vi "main_control_v1.vi"() -> ()   [LabVIEW 2021]
uses:
  Addons/DAQ_Pulse_Gen/DAQ_Control_2.ctl
  Addons/DAQ_Pulse_Gen/DAQ_Control_1.ctl
  Ver_2/Config_File_Paths_v2.ctl
  Ver_2/ZI_Data_v2.ctl
  Addons/DAQ_Pulse_Gen/DAQ_Control_3 .ctl
  <vilib>/Utility/file.llb/Write Delimited Spreadsheet (DBL).vi
  <vilib>/gmath/NumericalOptimization/Nonlinear Curve Fit LM formula string.vi
  <vilib>/Utility/Data Type/NI_Data Type.lvlib
  <vilib>/Analysis/NI_AALPro.lvlib
  <vilib>/gmath/NI_Gmath.lvlib
panel:
  out "tomography rotation memory (priv)":cluster{"Time":dbl[], dbl[]}[](array[cluster])
  in  "pulses type (priv)":string[](array[string])=["None", "Y pi/2", "X pi/2"]
  in  "stop":bool
  in  "Tab Control":T1(tab)=enum."Run single FID"
  out "Config folder":string
  out "Chennel names\nare correct (?)":bool
  out "Channel map":map{string, i32}(c390)
  out "Pulses map [us]":map{string, dbl}(c390)
  out "Sampling data":T2={"Sample Numbers"=20000000, "Sample  Frequency (Hz)"=20000000}
  out "Resource Address":T3={"ZI Address"="DEV714", "VISA Keithley"="KEITHLEY"}
  in  "Run tomography":bool
  in  "Run single FID":bool
  in  "Save for tomography":bool
  in  "Save single sequence":bool
  out "Pulses chart":cluster{dbl[], dbl[]}[](graph)
  in  "Reset sequence":bool
  in  "Channel":u16(ring) items=["LD pump", "LD repump", "LD probe", "pulse X", "pulse Y", "pulse Z", "Keithley ARM", "Keithley TRIG", "Accqusition TRIG", "Nonlinear coil", "None"]
  in  "Add pulse advanced":bool
  in  "Physical channels":string[](array[string])
  in  "Add pulse":bool
  in  "Time [us]":dbl
  in  "Z pi/2":bool
  in  "Z pi":bool
  in  "Y pi/2":bool
  in  "Y pi":bool
  in  "X pi/2":bool
  in  "X pi":bool
  in  "Add pumping":bool
  in  "Pumping":T4(ring)
  in  "save":bool
  out "Rotation signal 3":cluster{"Time":dbl[], "Array":dbl[]}[](graph)
  out "w":dbl format="%#_3f"
  out "q":dbl format="%#_3f"
  out "g2":dbl format="%#_3f"
  out "g1":dbl format="%#_3f"
  out "C":dbl format="%#_3f"
  out "B":dbl format="%#_3f"
  out "A":dbl format="%#_3f"
  in  "Enum":T5(ring)
  in  "Fit model":bool
  out "Rotation signal":cluster{"Time":dbl[], dbl[]}(graph)
  out "Rotation spectrum":waveform(dbl)[](graph)
  out "Differential signal":cluster{"Time":dbl[], "X":dbl[]}[](graph)
  out "Intensity signal":cluster{"Time":dbl[], dbl[]}(graph)
  out "Polarimeter":dbl(knob) scale=-10.0..10.0
  in  "Run single FID 2":bool
  out "Progress":dbl(slide) scale=0.0..100.0
  in  "Number of repetition":u32=1 min=1 step=1
  in  "Signal in X or Y (?)":bool
  in  "Plot type":u16(ring) items=["None + [ None ]", "None + [ Y pi ]", "None + [ Z(pi/2)+Y(pi) ]", "Y pi/2 + [ None ]", "Y pi/2 + [ Y pi ]", "Y pi/2 + [ Z(pi/2)+Y(pi) ]", "X pi/2 + [ None ]", "X pi/2 + [ Y pi ]", "X pi/2 + [ Z(pi/2)+Y(pi) ]"]
  in  "Save raw data (?)":bool
  in  "Save CYCLOPS data (?)":bool
  out "Rotation signal":cluster{"Time":dbl[], dbl[]}(graph)
  in  "Run tomography 2":bool
  in  "Averaging":u8=1 min=1 step=1
  out "Differential signal":cluster{"Time":dbl[], "X":dbl[]}[](graph)
  out "Intensity signal":cluster{"Time":dbl[], dbl[]}(graph)
  out "Progress":dbl(slide) scale=0.0..100.0
  out "Rotation spectrum":waveform(dbl)[](graph)
  out "Rotation":cluster{"Time":dbl[], dbl[]}(graph)
  # "To change that tab you need to go to block diagram"
  # "Probing will be added during saving"
  # "X"
  # "Y"
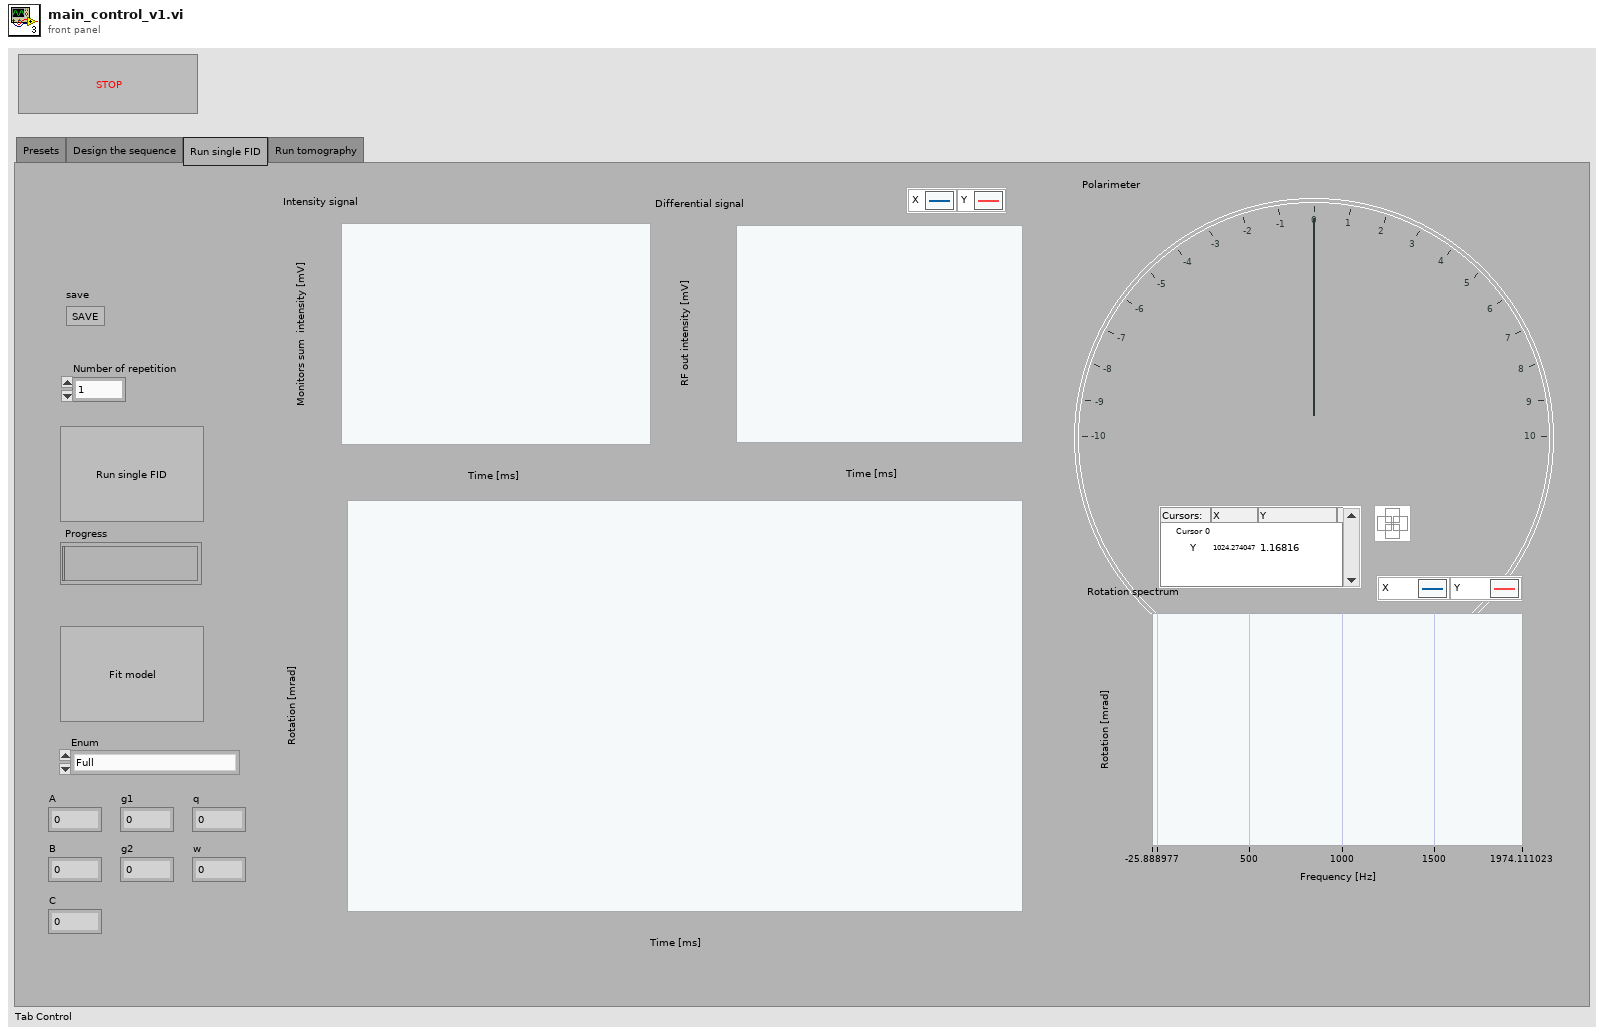
[diagram p1: front panel]
types:
  T1 = enum32{"Presets", "Design the sequence", "Run single FID", "Run tomography"}
  T2 = typedef "DAQ_Control_2.ctl" = cluster{"Sample Numbers":u32, "Sample  Frequency (Hz)":u32}
  T3 = cluster{"ZI Address":string, "VISA Keithley":refnum<visa-resource-name>}
  T4 = enum16{"Circular along X", "Linear in Y", "Linear in Z"}
  T5 = enum16{"Full", "A*Sin(w*t+q)*Exp(-g1*t)+C", "B*Exp(-q2*t)+C"}
  T6 = typedef "DAQ_Control_1.ctl" = cluster{"Port 2/line 6":cluster{"Timing 22":dbl[]}, "Port 2/line 5":cluster{"Timing 21":dbl[]}, "Port 2/line 4":cluster{"Timing 20":dbl[]}, "Port 2/line 3":cluster{"Timing 19":dbl[]}, "Port 2/line 2":cluster{"Timing 18":dbl[]}, "Port 2/line 1":cluster{"Timing 17":dbl[]}, "Port 2/line 0":cluster{"Timing 16":dbl[]}, "Port 1/line 7":cluster{"Timing 15":dbl[]}, "Port 1/line 6":cluster{"Timing 14":dbl[]}, "Port 1/line 5":cluster{"Timing 13":dbl[]}, "Port 1/line 4":cluster{"Timing 12":dbl[]}, "Port 1/line 3":cluster{"Timing 11":dbl[]}, "Port 1/line 2":cluster{"Timing 10":dbl[]}, "Port 1/line 1":cluster{"Timing 9":dbl[]}, "Port 1/line 0":cluster{"Timing 8":dbl[]}, "Port 0/line 7":cluster{"Timing 7\n":dbl[]}, "Port 0/line 6":cluster{"Timing 6\n":dbl[]}, "Port 0/line 5":cluster{"Timing 5\n":dbl[]}, "Port 0/line 4":cluster{"Timing 4\n":dbl[]}, "Port 0/line 3":cluster{"Timing 3\n":dbl[]}, "Port 0/line 2":cluster{"Timing 2":dbl[]}, "Port 0/line 1":cluster{"Timing 1\n":dbl[]}, "Port 0/line 0":cluster{"Timing 0":dbl[]}}
  T7 = typedef "Config_File_Paths_v2.ctl" = cluster{"ZI config file (.ini)":string, "Keithley config file (.ini)":string, "DAQ config file (.ini)":string}
  T8 = enum32{"Presets", "Design the sequence", "Run single FID"}
  T9 = enum8{"Enabled", "Disabled", "Disabled and Grayed Out"}
  T10 = cluster{"model":string, "Parameters":string[], "x":string}
  T11 = typedef "DAQ_Control_3 .ctl" = cluster{"Time Unit":enum16{"NanoSecond", "MicroSecond", "MilliSecond"}}
  T12 = typedef "ZI_Data_v2.ctl" = cluster{"R":dbl[], "Theta":dbl[], "X":dbl[], "Y":dbl[], "AuxIn0":dbl[], "AuxIn1":dbl[], "Frequency":dbl[], "DIO":dbl[], "Time":dbl[]}
  T13 = typedef "Resources_v2.ctl" = cluster{"ZI Handle":T14, "ZI ModHandle":T15, "VISA Keithley":refnum<visa-resource-name>}
  T14 = typedef "Zurich Instruments LabOne.lvlib/ziTypeHandle.ctl" = cluster{"handleValid":bool, "Conn":u64, "Path Prefix":string, "Handle":u64, "Connected":bool, "Clockbase(s)":dbl}
  T15 = typedef "Zurich Instruments LabOne.lvlib/ziTypeModHandle.ctl" = cluster{"handleValid":bool, "Conn":u64, "ModHandle":u64, "moduleID":string, "Path Prefix":string}
  T16 = typedef "Cutted_Data_v2.ctl" = cluster{"X":dbl[], "Y":dbl[], "Time":dbl[]}
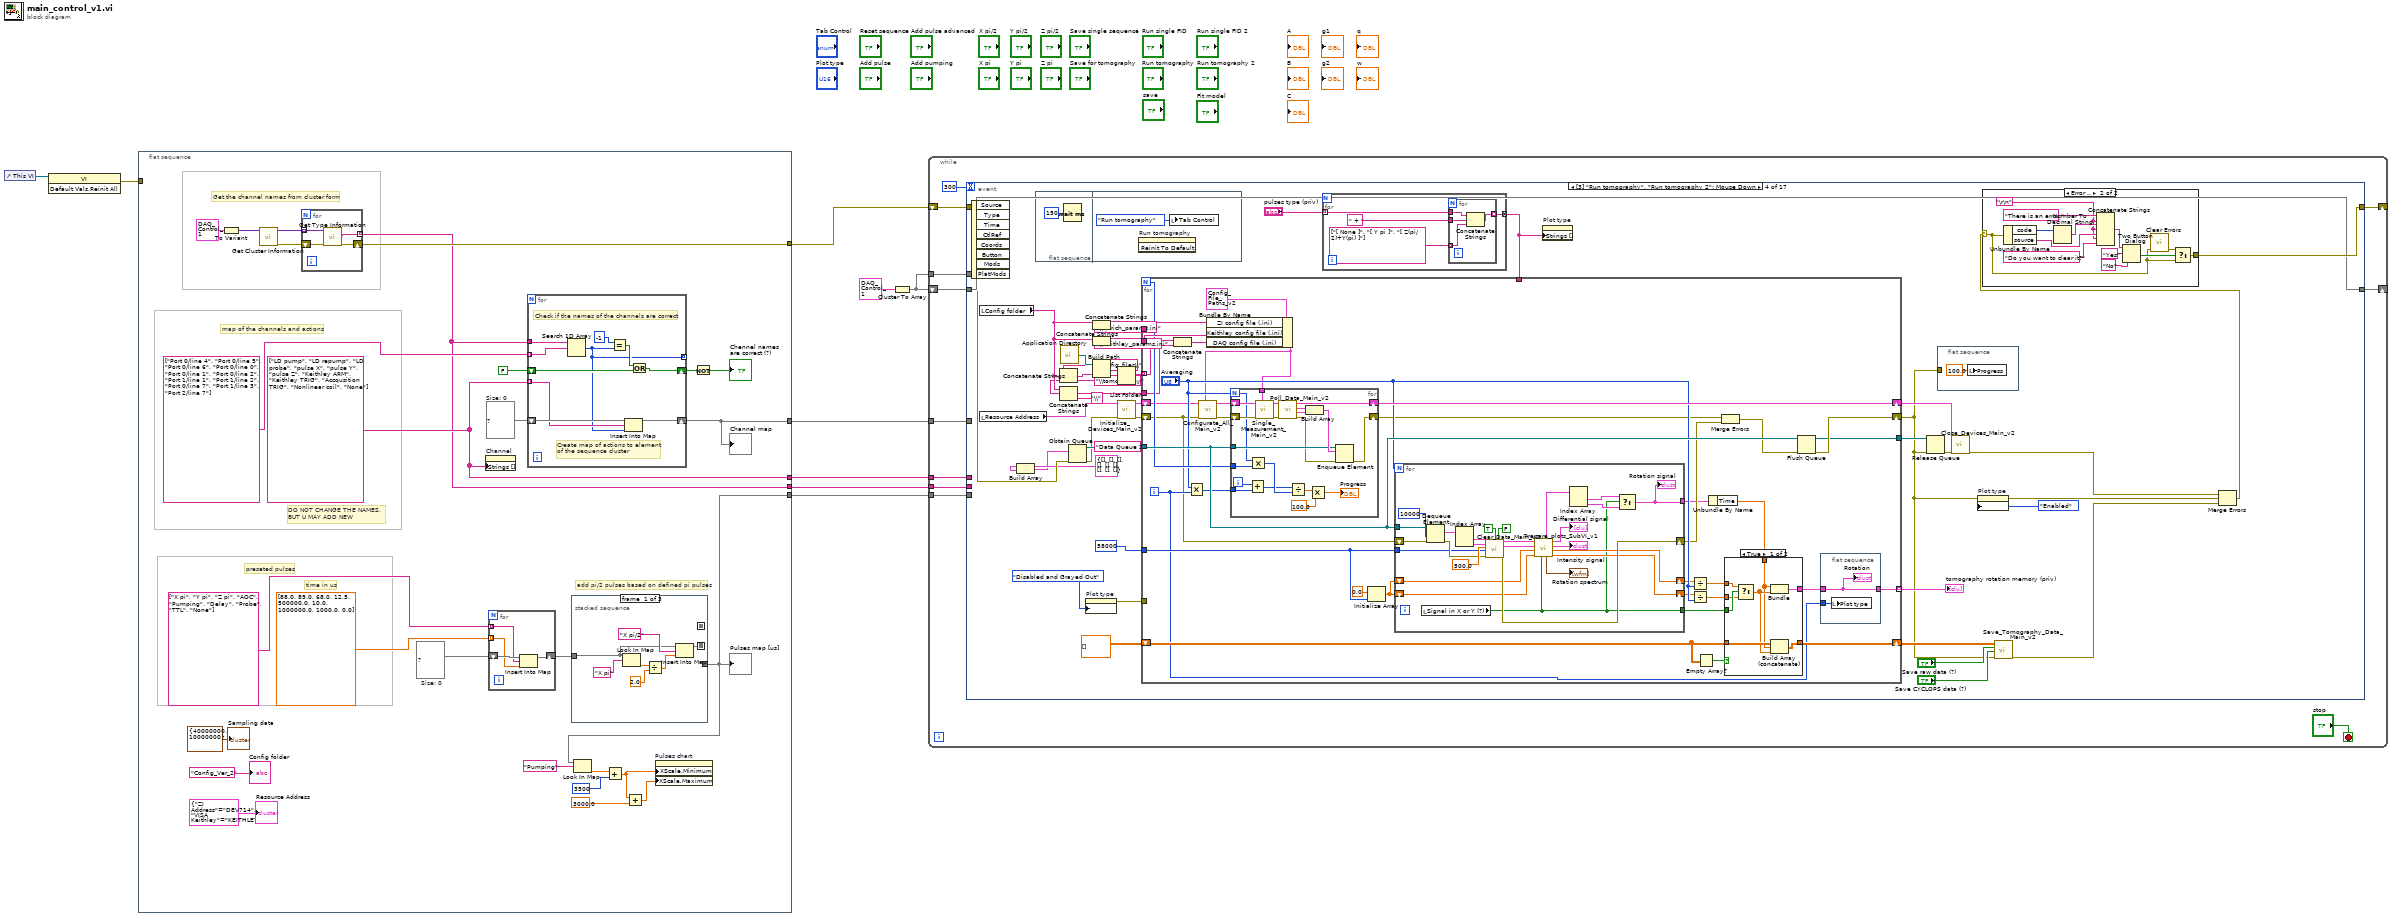
[diagram p0: block diagram]
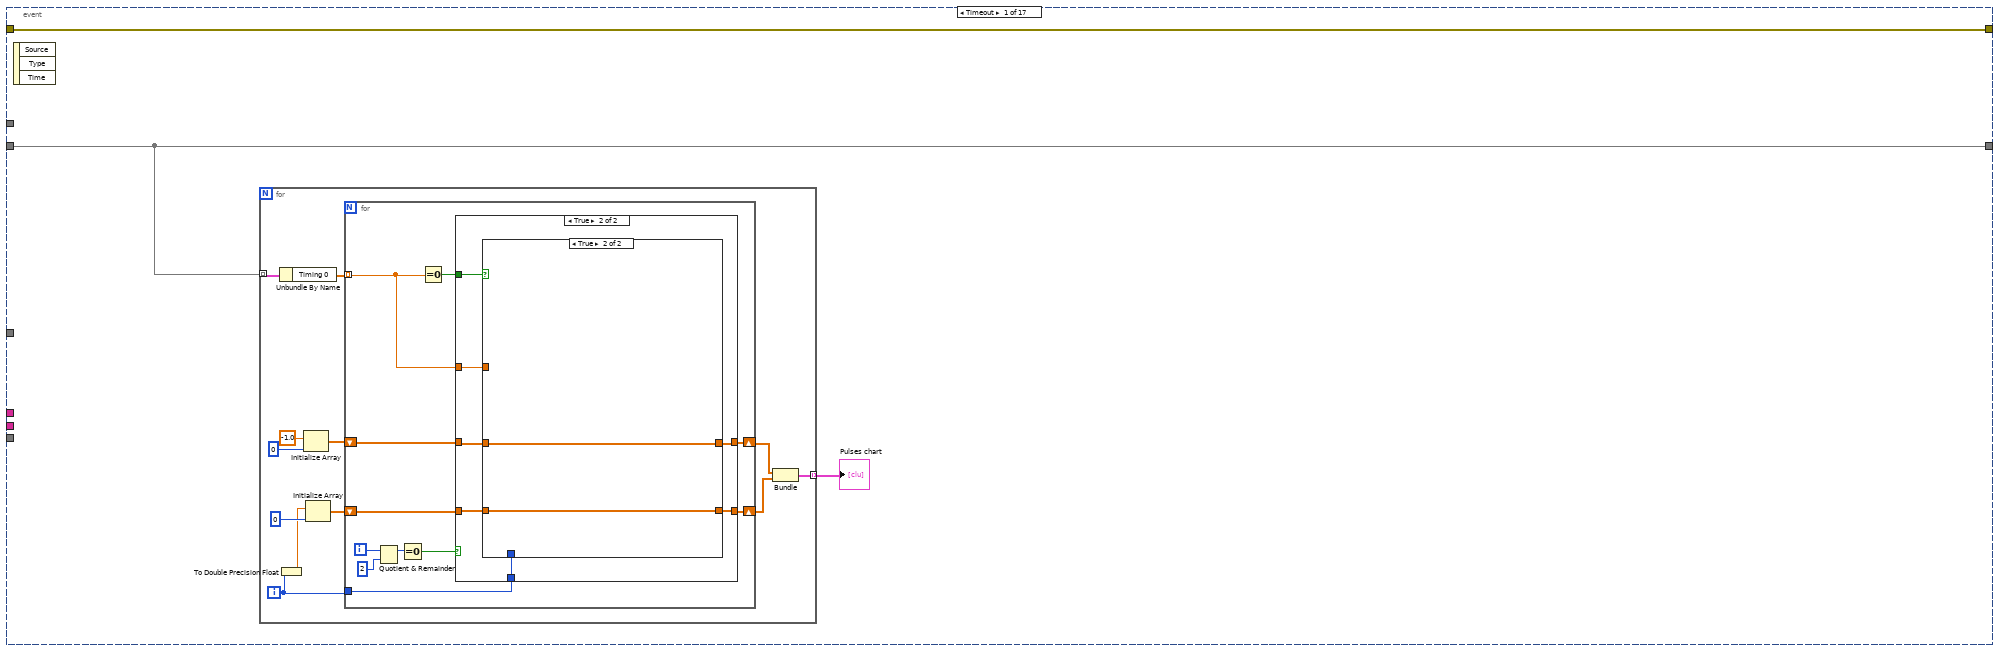
[diagram p2: hidden frame]
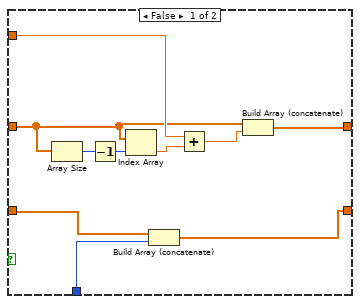
[diagram p3: hidden frame]
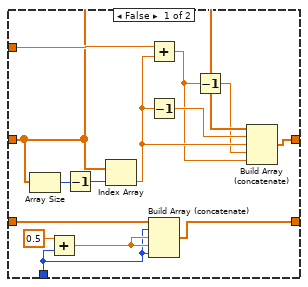
[diagram p4: hidden frame]
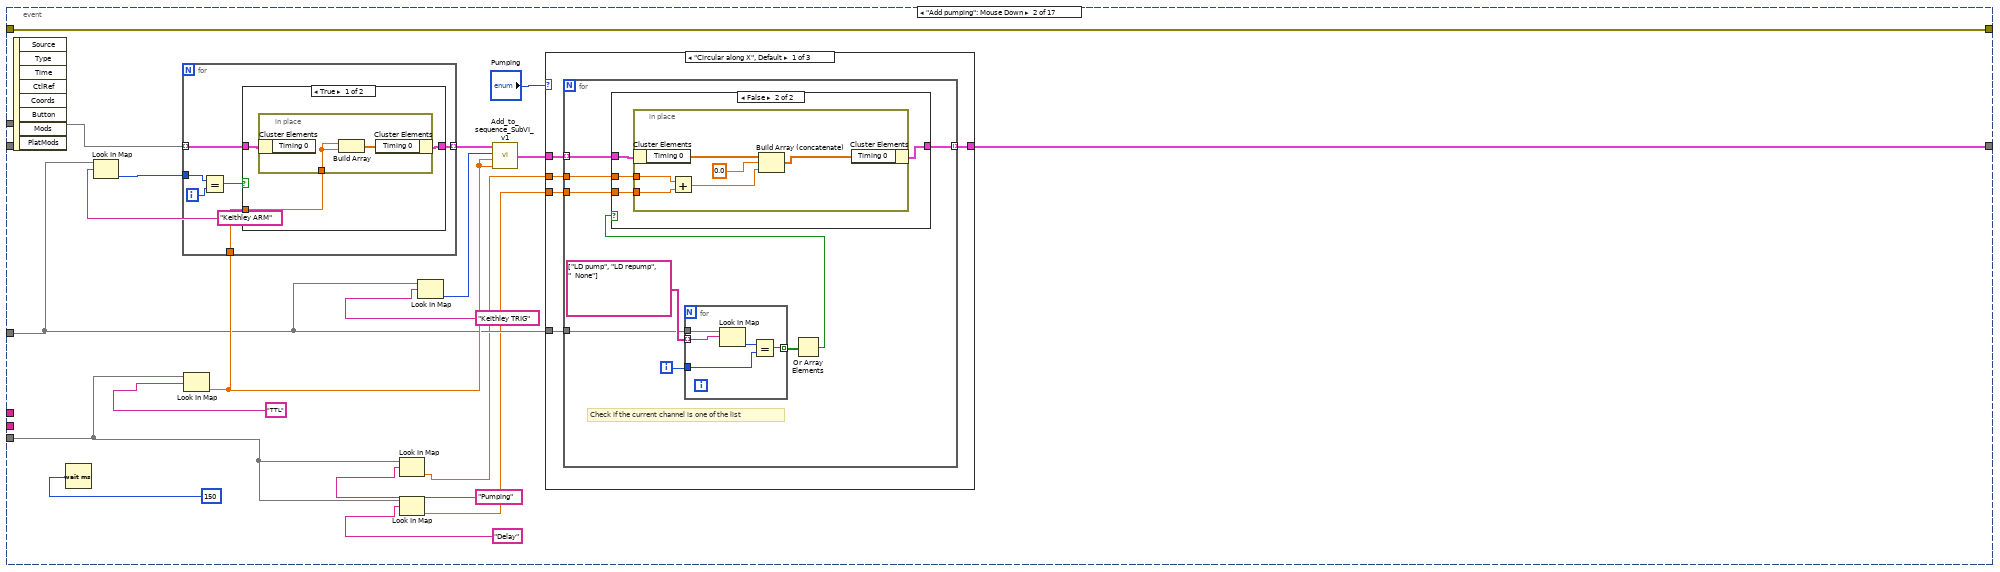
[diagram p5: hidden frame]
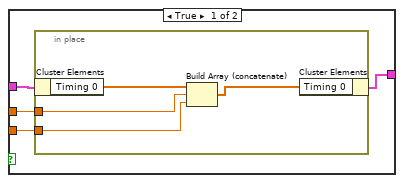
[diagram p6: hidden frame]
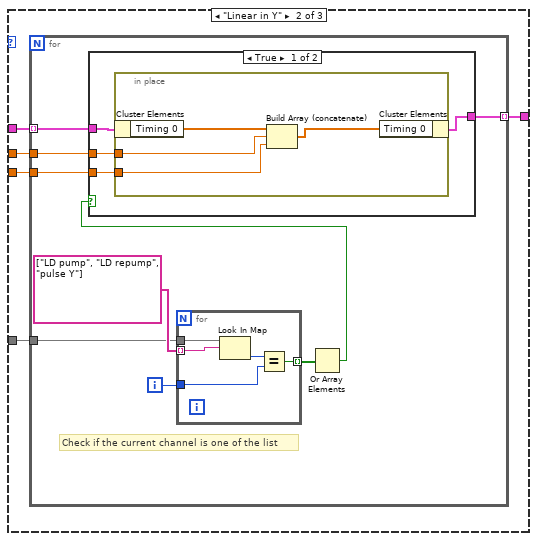
[diagram p7: hidden frame]
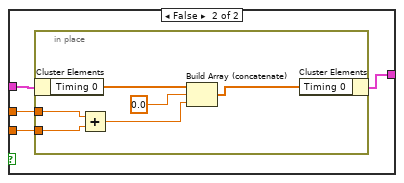
[diagram p8: hidden frame]
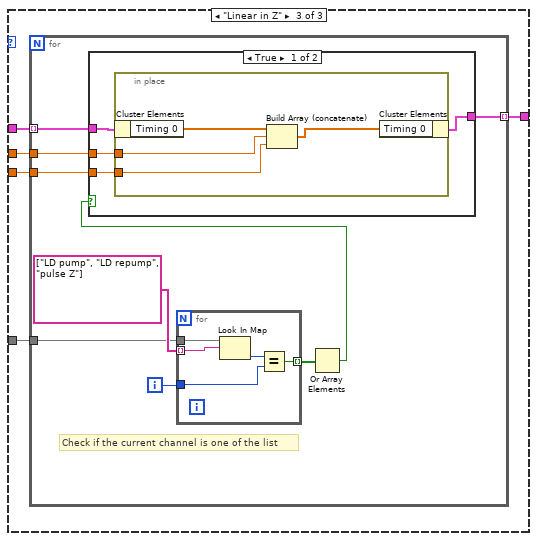
[diagram p9: hidden frame]
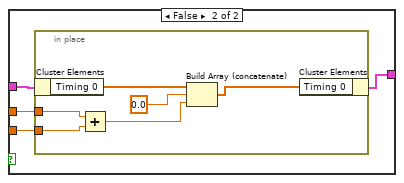
[diagram p10: hidden frame]
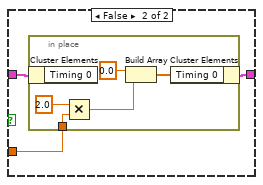
[diagram p11: hidden frame]
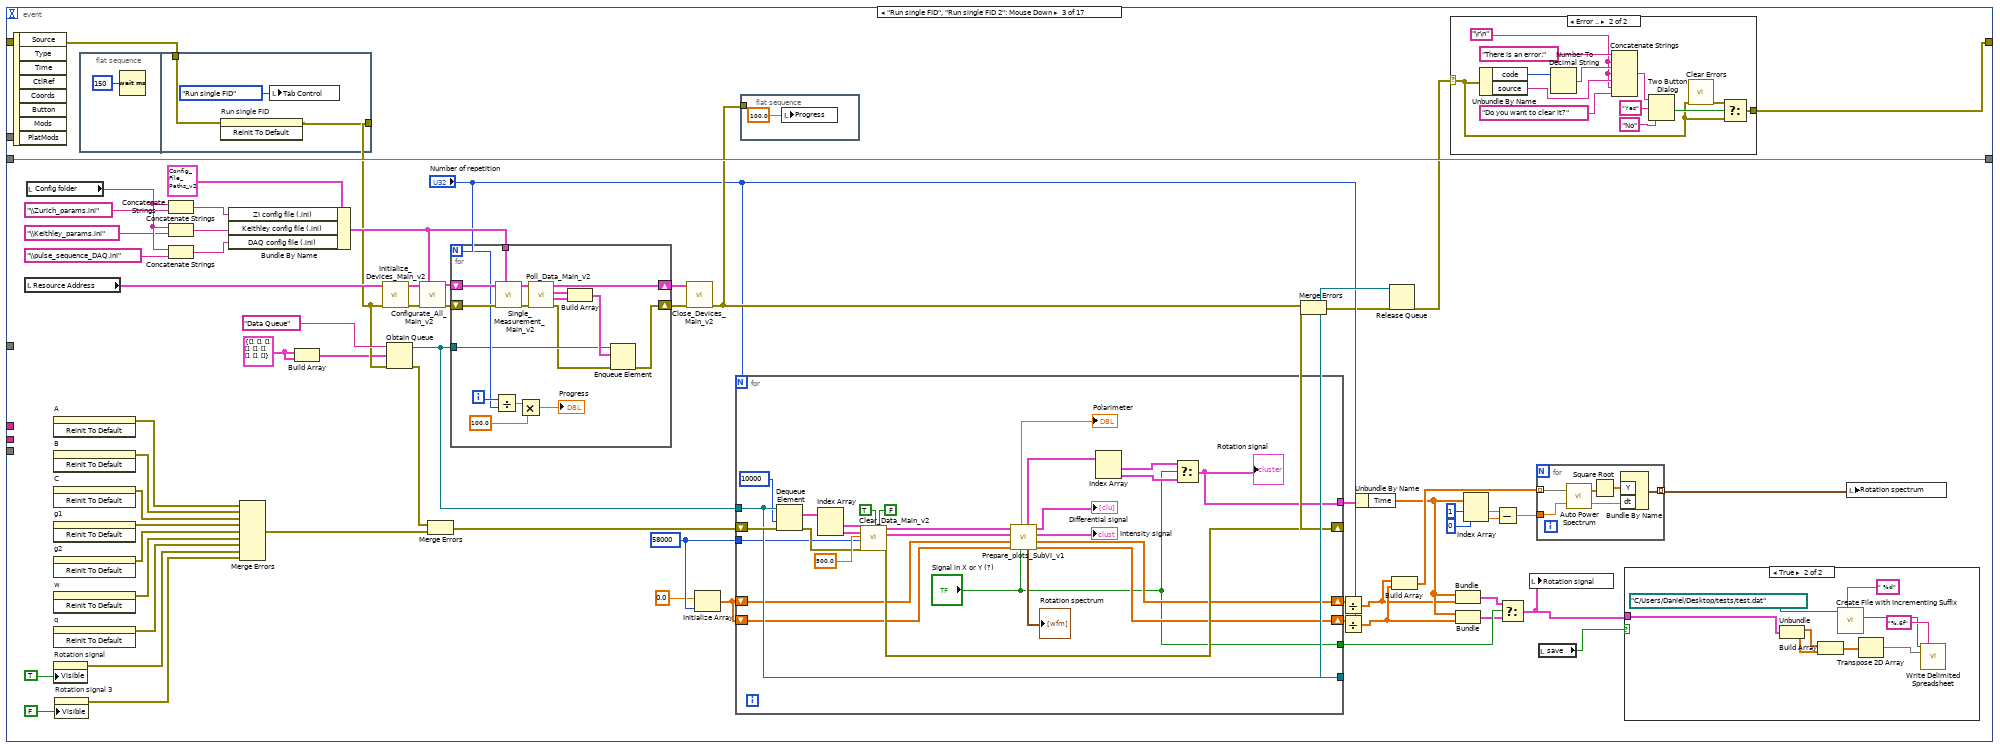
[diagram p12: hidden frame]
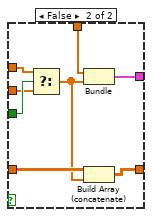
[diagram p15: hidden frame]
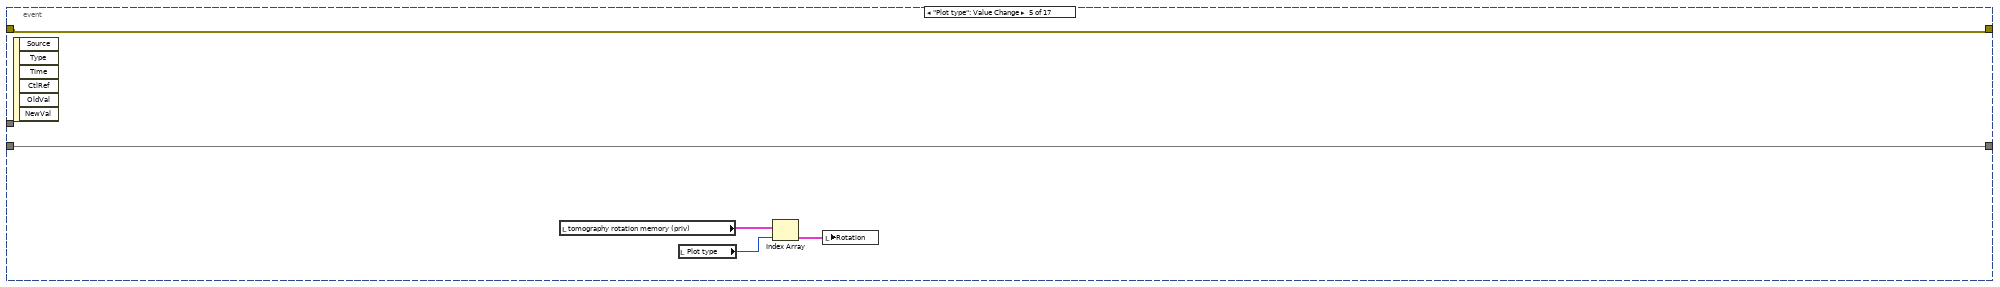
[diagram p17: hidden frame]
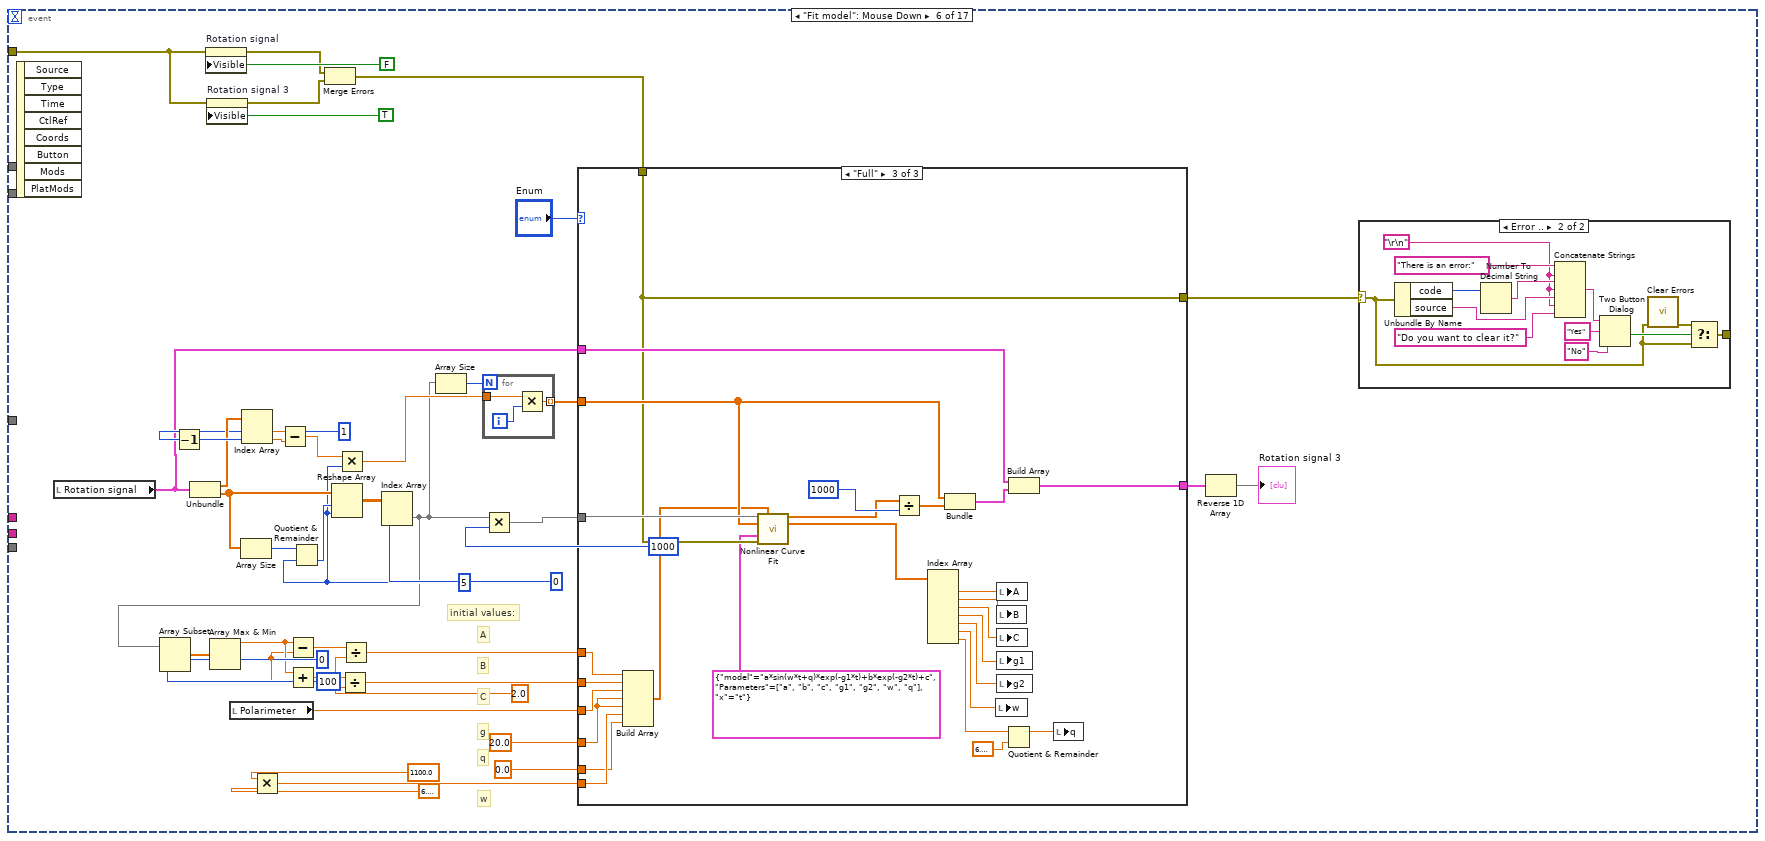
[diagram p18: hidden frame]
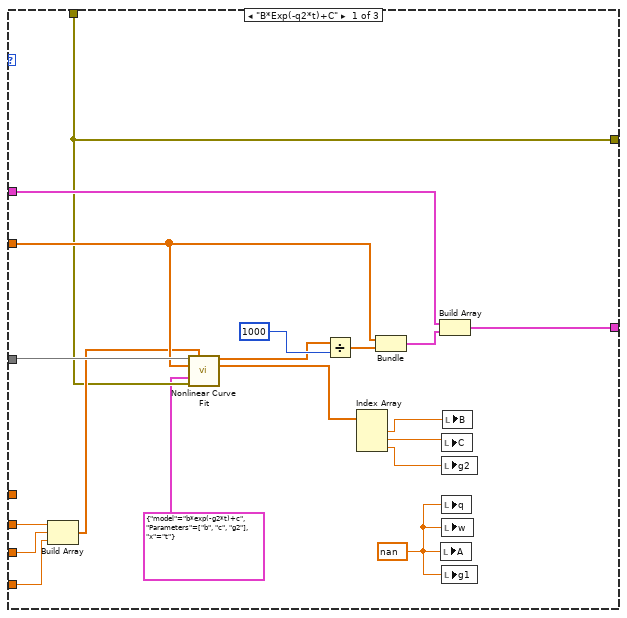
[diagram p20: hidden frame]
diagram:
  n1 = control-ref of="This VI"() -> (w2:refnum<vi>)
  n2 = invoke class="VI" method="Default Vals.Reinit All"(reference=w2) -> (error out=w1:errorcluster)  [unwired: 2 in, 2 out]
  n3 = flat-sequence {
    tunnel: [w23] -> w8
    tunnel: [w17] -> w7
    tunnel: [w22] -> w6
    tunnel: [w21] -> w5
    tunnel: [w20] -> w4
    tunnel: w1 -> [_]
    frame #0 {
      w27 = map{string, dbl} {}  # Size: 0
      w29 = map{string, i32} {}  # Size: 0
      w21 = string[] ["LD pump", "LD repump", "LD probe", "pulse X", "pulse Y", "pulse Z", "Keithley ARM", "Keithley TRIG", "Accqusition TRIG", "Nonlinear coil", "None"]
      # "DO NOT CHANGE THE NAMES,\nBUT U MAY ADD NEW"
      # "add pi/2 pulses based on defined pi pulses"
      # "preseted pulses"
      # "time in us"
      # "map of the channels and actions"
      # "Get the channel names from cluster form"
      n4 = To Variant(anything=T6 {"Port 2/line 6"={"Timing 22"=[]}, "Port 2/line 5"={"Timing 21"=[]}, "Port 2/line 4"={"Timing 20"=[]}, "Port 2/line 3"={"Timing 19"=[]}, "Port 2/line 2"={"Timing 18"=[]}, "Port 2/line 1"={"Timing 17"=[]}, "Port 2/line 0"={"Timing 16"=[]}, "Port 1/line 7"={"Timing 15"=[]}, "Port 1/line 6"={"Timing 14"=[]}, "Port 1/line 5"={"Timing 13"=[]}, "Port 1/line 4"={"Timing 12"=[]}, "Port 1/line 3"={"Timing 11"=[]}, "Port 1/line 2"={"Timing 10"=[]}, "Port 1/line 1"={"Timing 9"=[]}, "Port 1/line 0"={"Timing 8"=[]}, "Port 0/line 7"={"Timing 7\n"=[]}, "Port 0/line 6"={"Timing 6\n"=[]}, "Port 0/line 5"={"Timing 5\n"=[]}, "Port 0/line 4"={"Timing 4\n"=[]}, "Port 0/line 3"={"Timing 3\n"=[]}, "Port 0/line 2"={"Timing 2"=[]}, "Port 0/line 1"={"Timing 1\n"=[]}, "Port 0/line 0"={"Timing 0"=[]}} ("Sequence")) -> (Variant=w35:variant)
      n5 = call <vilib>:"Get Cluster Information.vi"("variant"=w35) -> ("error out"=w34:errorcluster, "cluster elements"=w33:variant[])  [unwired: 9 in]
      n6 = for {
        tunnel: w33 -> [w75] mode=indexing
        shift-right: [w73] -> w22
        shift-left: w34 -> [w74]
        tunnel: [w72] -> w20 mode=indexing
        n7 = call <vilib>:"Get Type Information.vi"("error in (no error)"=w74, "variant"=w75) -> ("error out"=w73:errorcluster, "name"=w72:string)  [unwired: 5 in, 3 out]
      }
      n8 = property on="Channel" class="Ring (strict)"("Strings []"=w21) -> ()  [unwired: 2 in, 2 out]
      n9 = for {
        shift-right: [w58] -> w24
        shift-left: w27 -> [w61]
        tunnel: string[] ["X pi", "Y pi", "Z pi", "AOC", "Pumping", "Delay", "Probe", "TTL", "None"] -> [w60] mode=indexing
        tunnel: dbl[] [88.0, 89.0, 68.0, 12.5, 500000.0, 10.0, 1000000.0, 1000.0, 0.0] -> [w59] mode=indexing
        n10 = Insert Into Map(map in=w61, key=w60, value=w59) -> (map out=w58:map{string, dbl})  [unwired: 2 out]
      }
      n11 = for {
        tunnel: w20 -> [w71]
        tunnel: string[] ["Port 0/line 4", "Port 0/line 5", "Port 0/line 6", "Port 0/line 0", "Port 0/line 1", "Port 0/line 2", "Port 1/line 1", "Port 1/line 2", "Port 0/line 7", "Port 1/line 3", "Port 2/line 7"] -> [w62] mode=indexing
        shift-right: [w67] -> w31
        shift-left: FALSE -> [w68]
        tunnel: [w64] -> _ mode=indexing
        shift-right: [w63] -> w23
        shift-left: w29 -> [w66]
        tunnel: w21 -> [w65] mode=indexing
        # "Create map of actions to element\nof the sequence cluster"
        # "Check if the names of the channels are correct"
        n12 = Search 1D Array(1D array=w71, element=w62) -> (index of element=w64:i32)  [unwired: 1 in]
        n13 = Equal?(x=-1, y=w64) -> (x = y?=w69:bool)
        n14 = Insert Into Map(map in=w66, key=w65, value=w64) -> (map out=w63:map{string, i32})  [unwired: 2 out]
        n15 = Or(x=w69, y=w68) -> (x .or. y?=w67:bool)
      }
      "Channel map" <- w23
      n16 = stacked-sequence {
        seq-local: [w37 _ _] -> [_ w44 _]
        seq-local: [_ w45 _] -> [_ _ w52]
        tunnel: w24 -> [w41 _ _]
        tunnel: [_ _ w51] -> w17
        frame #0 {
          n17 = Look In Map(map=w41, key="X pi") -> (value=w39:dbl)  [unwired: 1 in, 1 out]
          n18 = Divide(x=w39, y=2.0) -> (x/y=w40:dbl)
          n19 = Insert Into Map(map in=w41, key="X pi/2", value=w40) -> (map out=w37:map{string, dbl})  [unwired: 2 out]
        }
        frame #1 {
          n20 = Look In Map(map=w44, key="Y pi") -> (value=w50:dbl)  [unwired: 1 in, 1 out]
          n21 = Divide(x=w50, y=2.0) -> (x/y=w49:dbl)
          n22 = Insert Into Map(map in=w44, key="Y pi/2", value=w49) -> (map out=w45:map{string, dbl})  [unwired: 2 out]
        }
        frame #2 {
          n23 = Look In Map(map=w52, key="Z pi") -> (value=w54:dbl)  [unwired: 1 in, 1 out]
          n24 = Divide(x=w54, y=2.0) -> (x/y=w55:dbl)
          n25 = Insert Into Map(map in=w52, key="Z pi/2", value=w55) -> (map out=w51:map{string, dbl})  [unwired: 2 out]
        }
      }
      "Pulses map [us]" <- w17
      n26 = Look In Map(map=w17, key="Pumping") -> (value=w19:dbl)  [unwired: 1 in, 1 out]
      n27 = Add(x=w19, y=3500) -> (x+y=w16:dbl)
      n28 = Add(x=w16, y=3000.0) -> (x+y=w14:dbl)
      n29 = property on="Pulses chart" class="XYGraph (strict)"("XScale.Minimum"=w16, "XScale.Maximum"=w14) -> ()  [unwired: 2 in, 2 out]
      n30 = Not(x=w31) -> (.not. x?=→"Chennel names\nare correct (?)":bool)
      "Sampling data" <- T2 {"Sample Numbers"=40000000, "Sample  Frequency (Hz)"=10000000} ("Sampling data")
      "Config folder" <- "Config_Ver_2" ("Filename (ini)")
      "Resource Address" <- T3 {"ZI Address"="DEV714", "VISA Keithley"="KEITHLEY"} ("Resource Address")
    }
  }
  n31 = Cluster To Array(cluster=T6 {"Port 2/line 6"={"Timing 22"=[]}, "Port 2/line 5"={"Timing 21"=[]}, "Port 2/line 4"={"Timing 20"=[]}, "Port 2/line 3"={"Timing 19"=[]}, "Port 2/line 2"={"Timing 18"=[]}, "Port 2/line 1"={"Timing 17"=[]}, "Port 2/line 0"={"Timing 16"=[]}, "Port 1/line 7"={"Timing 15"=[]}, "Port 1/line 6"={"Timing 14"=[]}, "Port 1/line 5"={"Timing 13"=[]}, "Port 1/line 4"={"Timing 12"=[]}, "Port 1/line 3"={"Timing 11"=[]}, "Port 1/line 2"={"Timing 10"=[]}, "Port 1/line 1"={"Timing 9"=[]}, "Port 1/line 0"={"Timing 8"=[]}, "Port 0/line 7"={"Timing 7\n"=[]}, "Port 0/line 6"={"Timing 6\n"=[]}, "Port 0/line 5"={"Timing 5\n"=[]}, "Port 0/line 4"={"Timing 4\n"=[]}, "Port 0/line 3"={"Timing 3\n"=[]}, "Port 0/line 2"={"Timing 2"=[]}, "Port 0/line 1"={"Timing 1\n"=[]}, "Port 0/line 0"={"Timing 0"=[]}} ("Sequence")) -> (array=w3:cluster{"Timing 0":dbl[]}[])
  n32 = while {
    shift-right: [w77] -> _
    shift-left: w3 -> [w86]
    tunnel: w8 -> [w85]
    tunnel: w7 -> [w76]
    shift-right: [w81] -> _
    shift-left: w6 -> [w82]
    tunnel: w5 -> [w80]
    tunnel: w4 -> [w79]
    tunnel: w3 -> [w78]
    stop <- "stop" stop-if-true
    n33 = event shown="[3] \"Run tomography\", \"Run tomography 2\": Mouse Down" {
      selector: _ -> [_ _ _ _ _ _ _ _ _ _ _ _ _ _ _ _ _]
      dyn-events: _ -> [_ _ _ _ _ _ _ _ _ _ _ _ _ _ _ _ _]
      timeout: 300 -> [_ _ _ _ _ _ _ _ _ _ _ _ _ _ _ _ _]
      tunnel: w86 -> [w89 _ w343 w472 w608 _ w750 w762 w774 w786 w798 w810 w822 w845 w884 w955 _]
      tunnel: w85 -> [_ w151 _ _ _ _ w757 w769 w781 w793 w805 w817 w828 _ w897 w960 _]
      tunnel: w76 -> [_ w150 _ _ _ _ w751 w763 w775 w787 w799 w811 w823 w837 w894 w959 _]
      tunnel: [w89 w148 w343 w472 w608 _ w749 w761 w773 w785 w797 w809 w821 w834 w884 w955 w1097] -> w77
      tunnel: w82 -> [w88 w164 w342 w466 w609 w651 w753 w765 w777 w789 w801 w813 w826 w841 w879 w953 w1098]
      tunnel: [w88 w164 w321 w476 w609 _ w753 w765 w777 w789 w801 w813 w826 w841 w878 w952 w1098] -> w81
      tunnel: w80 -> [_ _ _ _ _ _ _ _ _ _ _ _ w829 _ _ _ _]
      tunnel: w79 -> [_ _ _ _ _ _ _ _ _ _ _ _ _ w843 _ _ _]
      tunnel: w78 -> [_ w147 _ _ _ _ _ _ _ _ _ _ _ _ _ _ w1097]
      event Timeout {
        n34 = event-data() -> ()  [unwired: 1 in, 3 out]
        n35 = for {
          tunnel: w89 -> [w101] mode=indexing
          tunnel: [w90] -> w87 mode=indexing
          i -> [w93]
          n36 = To Double Precision Float(number=w93) -> (double precision float=w97:dbl)
          n37 = Unbundle By Name(w101) -> ("Timing 0"=w100:dbl[])
          n38 = Initialize Array(-1.0 ("element"), 0 ("dimension size")) -> (w94:dbl[])
          n39 = Initialize Array(w97, 0 ("dimension size")) -> (w98:dbl[])
          n40 = for {
            tunnel: w100 -> [w103] mode=indexing
            shift-right: [w105] -> w91
            shift-left: w98 -> [w104]
            shift-right: [w107] -> w92
            shift-left: w94 -> [w106]
            tunnel: w93 -> [w102]
            i -> [w112]
            n41 = Quotient & Remainder(x=w112, y=2) -> (x-y*floor(x/y)=w110:i32)  [unwired: 1 out]
            n42 = Equal To 0?(x=w110) -> (x = 0?=w109:bool)
            n43 = Equal To 0?(x=w103) -> (x = 0?=w108:bool)
            n44 = case shown="True" w109 {
              tunnel: w108 -> [_ w129]
              tunnel: [w113 w128] -> w107
              tunnel: w106 -> [w115 w127]
              tunnel: [w120 w126] -> w105
              tunnel: w104 -> [w121 w125]
              tunnel: w103 -> [w116 w124]
              tunnel: w102 -> [w122 w123]
              frame False {
                n45 = Array Size(array=w115) -> (size(s)=w119:i32)
                n46 = Decrement(x=w119) -> (x-1=w118:i32)
                n47 = Index Array(array=w115, index=w118) -> (element=w117:dbl)
                n48 = Build Array (concatenate)(w121, w122) -> (w120:dbl[])
                n49 = Add(x=w116, y=w117) -> (x+y=w114:dbl)
                n50 = Build Array (concatenate)(w115, w114) -> (w113:dbl[])
              }
              frame True {
                n51 = case shown="True" w129 {
                  tunnel: [w140 w145] -> w128
                  tunnel: w127 -> [w134 w145]
                  tunnel: [w136 w144] -> w126
                  tunnel: w125 -> [w143 w144]
                  tunnel: w124 -> [w141 _]
                  tunnel: w123 -> [w137 _]
                  frame False {
                    n52 = Array Size(array=w134) -> (size(s)=w142:i32)
                    n53 = Add(x=0.5, y=w137) -> (x+y=w138:dbl)
                    n54 = Decrement(x=w142) -> (x-1=w135:i32)
                    n55 = Index Array(array=w134, index=w135) -> (element=w132:dbl)
                    n56 = Add(x=w141, y=w132) -> (x+y=w131:dbl)
                    n57 = Decrement(x=w132) -> (x-1=w133:dbl)
                    n58 = Build Array (concatenate)(w143, w137, w138, w138, w137) -> (w136:dbl[])
                    n59 = Decrement(x=w131) -> (x-1=w130:dbl)
                    n60 = Build Array (concatenate)(w134, w133, w132, w130, w131) -> (w140:dbl[])
                  }
                  frame True {
                  }
                }
              }
            }
          }
          n61 = Bundle(w92, w91) -> (w90:cluster{dbl[], dbl[]})  [unwired: 1 in]
        }
        "Pulses chart" <- w87
      }
      event "Add pumping": Mouse Down {
        n62 = event-data() -> ()  [unwired: 1 in, 8 out]
        n63 = Wait (ms)(milliseconds to wait=u32 150) -> ()  [unwired: 1 out]
        n64 = Look In Map(map=w151, key="Keithley ARM") -> (value=w161:i32)  [unwired: 1 in, 1 out]
        n65 = Look In Map(map=w150, key="TTL") -> (value=w156:dbl)  [unwired: 1 in, 1 out]
        n66 = for {
          tunnel: w147 -> [w278] mode=indexing
          tunnel: w161 -> [w280]
          tunnel: w156 -> [w277]
          tunnel: [w276] -> w159 mode=indexing
          i -> [w281]
          n67 = Equal?(x=w280, y=w281) -> (x = y?=w279:bool)
          n68 = case shown="True" w279 {
            tunnel: w278 -> [w284 w289]
            tunnel: w277 -> [w283 w288]
            tunnel: [w282 w287] -> w276
            frame True {
              n69 = in-place {
                in-place-border: w283 -> [w286]
                n70 = in-place-cluster #1(w284) -> ()  [unwired: 1 out]
                n71 = Build Array(w286, w286) -> (w285:dbl[])
                n72 = in-place-cluster #1("Timing 0"=w285) -> (w282:cluster{"Timing 0":dbl[]})
              }
            }
            frame False {
              n73 = in-place {
                in-place-border: w288 -> [w292]
                n74 = in-place-cluster #2(w289) -> ()  [unwired: 1 out]
                n75 = Multiply(x=2.0, y=w292) -> (x*y=w290:dbl)
                n76 = Build Array(0.0 ("element"), w290) -> (w294:dbl[])
                n77 = in-place-cluster #2("Timing 0"=w294) -> (w287:cluster{"Timing 0":dbl[]})
              }
            }
          }
        }
        n78 = Look In Map(map=w150, key="Pumping") -> (value=w146:dbl)  [unwired: 1 in, 1 out]
        n79 = Look In Map(map=w150, key="Delay") -> (value=w149:dbl)  [unwired: 1 in, 1 out]
        n80 = Look In Map(map=w151, key="Keithley TRIG") -> (value=w157:i32)  [unwired: 1 in, 1 out]
        n81 = call "Add_to_sequence_SubVI_v1.vi"("Delay [us]"=w156, "Pulse length [us]"=w156, "Channel number"=w157, "Array sequence in"=w159) -> ("Array sequence out"=w154:cluster{"Timing 0":dbl[]}[])
        n82 = case shown="\"Circular along X\", Default" "Pumping" {
          tunnel: w154 -> [w169 w206 w243]
          tunnel: w151 -> [w168 w205 w242]
          tunnel: w146 -> [w167 w204 w241]
          tunnel: w149 -> [w166 w203 w240]
          tunnel: [w165 w202 w239] -> w148
          frame "Circular along X", Default {
            n83 = for {
              tunnel: w169 -> [w173] mode=indexing
              tunnel: w168 -> [w175]
              tunnel: w167 -> [w172]
              tunnel: w166 -> [w171]
              tunnel: [w170] -> w165 mode=indexing
              i -> [w176]
              # "Check if the current channel is one of the list"
              n84 = for {
                tunnel: w175 -> [w200]
                tunnel: w176 -> [w199]
                tunnel: [w198] -> w178 mode=indexing
                tunnel: string[] ["LD pump", "LD repump", "  None"] -> [w197] mode=indexing
                n85 = Look In Map(map=w200, key=w197) -> (value=w201:i32)  [unwired: 1 in, 1 out]
                n86 = Equal?(x=w201, y=w199) -> (x = y?=w198:bool)
              }
              n87 = Or Array Elements(Boolean array=w178) -> (logical OR=w174:bool)
              n88 = case shown="False" w174 {
                tunnel: w173 -> [w182 w190]
                tunnel: w172 -> [w181 w189]
                tunnel: w171 -> [w180 w188]
                tunnel: [w179 w187] -> w170
                frame True {
                  n89 = in-place {
                    in-place-border: w181 -> [w185]
                    in-place-border: w180 -> [w184]
                    n90 = in-place-cluster #3(w182) -> ("Timing 0"=w186:dbl[])
                    n91 = Build Array (concatenate)(w186, w185, w184) -> (w183:dbl[])
                    n92 = in-place-cluster #3("Timing 0"=w183) -> (w179:cluster{"Timing 0":dbl[]})
                  }
                }
                frame False {
                  n93 = in-place {
                    in-place-border: w189 -> [w194]
                    in-place-border: w188 -> [w193]
                    n94 = in-place-cluster #4(w190) -> ("Timing 0"=w196:dbl[])
                    n95 = Add(x=w194, y=w193) -> (x+y=w192:dbl)
                    n96 = Build Array (concatenate)(w196, 0.0 ("element"), w192) -> (w195:dbl[])
                    n97 = in-place-cluster #4("Timing 0"=w195) -> (w187:cluster{"Timing 0":dbl[]})
                  }
                }
              }
            }
          }
          frame "Linear in Y" {
            n98 = for {
              tunnel: w206 -> [w210] mode=indexing
              tunnel: w205 -> [w212]
              tunnel: w204 -> [w209]
              tunnel: w203 -> [w208]
              tunnel: [w207] -> w202 mode=indexing
              i -> [w213]
              # "Check if the current channel is one of the list"
              n99 = for {
                tunnel: w212 -> [w237]
                tunnel: w213 -> [w236]
                tunnel: [w235] -> w215 mode=indexing
                tunnel: string[] ["LD pump", "LD repump", "pulse Y"] -> [w234] mode=indexing
                n100 = Look In Map(map=w237, key=w234) -> (value=w238:i32)  [unwired: 1 in, 1 out]
                n101 = Equal?(x=w238, y=w236) -> (x = y?=w235:bool)
              }
              n102 = Or Array Elements(Boolean array=w215) -> (logical OR=w211:bool)
              n103 = case shown="True" w211 {
                tunnel: w210 -> [w219 w227]
                tunnel: w209 -> [w218 w226]
                tunnel: w208 -> [w217 w225]
                tunnel: [w216 w224] -> w207
                frame True {
                  n104 = in-place {
                    in-place-border: w218 -> [w222]
                    in-place-border: w217 -> [w221]
                    n105 = in-place-cluster #5(w219) -> ("Timing 0"=w223:dbl[])
                    n106 = Build Array (concatenate)(w223, w222, w221) -> (w220:dbl[])
                    n107 = in-place-cluster #5("Timing 0"=w220) -> (w216:cluster{"Timing 0":dbl[]})
                  }
                }
                frame False {
                  n108 = in-place {
                    in-place-border: w226 -> [w231]
                    in-place-border: w225 -> [w230]
                    n109 = in-place-cluster #6(w227) -> ("Timing 0"=w233:dbl[])
                    n110 = Add(x=w231, y=w230) -> (x+y=w229:dbl)
                    n111 = Build Array (concatenate)(w233, 0.0 ("element"), w229) -> (w232:dbl[])
                    n112 = in-place-cluster #6("Timing 0"=w232) -> (w224:cluster{"Timing 0":dbl[]})
                  }
                }
              }
            }
          }
          frame "Linear in Z" {
            n113 = for {
              tunnel: w243 -> [w247] mode=indexing
              tunnel: w242 -> [w249]
              tunnel: w241 -> [w246]
              tunnel: w240 -> [w245]
              tunnel: [w244] -> w239 mode=indexing
              i -> [w250]
              # "Check if the current channel is one of the list"
              n114 = for {
                tunnel: w249 -> [w274]
                tunnel: w250 -> [w273]
                tunnel: [w272] -> w252 mode=indexing
                tunnel: string[] ["LD pump", "LD repump", "pulse Z"] -> [w271] mode=indexing
                n115 = Look In Map(map=w274, key=w271) -> (value=w275:i32)  [unwired: 1 in, 1 out]
                n116 = Equal?(x=w275, y=w273) -> (x = y?=w272:bool)
              }
              n117 = Or Array Elements(Boolean array=w252) -> (logical OR=w248:bool)
              n118 = case shown="True" w248 {
                tunnel: w247 -> [w256 w264]
                tunnel: w246 -> [w255 w263]
                tunnel: w245 -> [w254 w262]
                tunnel: [w253 w261] -> w244
                frame True {
                  n119 = in-place {
                    in-place-border: w255 -> [w259]
                    in-place-border: w254 -> [w258]
                    n120 = in-place-cluster #7(w256) -> ("Timing 0"=w260:dbl[])
                    n121 = Build Array (concatenate)(w260, w259, w258) -> (w257:dbl[])
                    n122 = in-place-cluster #7("Timing 0"=w257) -> (w253:cluster{"Timing 0":dbl[]})
                  }
                }
                frame False {
                  n123 = in-place {
                    in-place-border: w263 -> [w268]
                    in-place-border: w262 -> [w267]
                    n124 = in-place-cluster #8(w264) -> ("Timing 0"=w270:dbl[])
                    n125 = Add(x=w268, y=w267) -> (x+y=w266:dbl)
                    n126 = Build Array (concatenate)(w270, 0.0 ("element"), w266) -> (w269:dbl[])
                    n127 = in-place-cluster #8("Timing 0"=w269) -> (w261:cluster{"Timing 0":dbl[]})
                  }
                }
              }
            }
          }
        }
      }
      event "Run single FID", "Run single FID 2": Mouse Down {
        w303 = T12 {"R"=[], "Theta"=[], "X"=[], "Y"=[], "AuxIn0"=[], "AuxIn1"=[], "Frequency"=[], "DIO"=[], "Time"=[]} ("ZI Data")
        w337 = u16 58000 ("Fixed Number Of Points")
        n128 = event-data() -> ()  [unwired: 1 in, 8 out]
        n129 = local read "Resource Address"() -> (w359:T3)
        n130 = local read "Config folder"() -> (w356:string)
        n131 = invoke on="A" class="DigNum (strict)" method="Reinit To Default"() -> (error out=w311:errorcluster)  [unwired: 3 in, 2 out]
        n132 = invoke on="B" class="DigNum (strict)" method="Reinit To Default"() -> (error out=w312:errorcluster)  [unwired: 3 in, 2 out]
        n133 = invoke on="C" class="DigNum (strict)" method="Reinit To Default"() -> (error out=w313:errorcluster)  [unwired: 3 in, 2 out]
        n134 = invoke on="g1" class="DigNum (strict)" method="Reinit To Default"() -> (error out=w314:errorcluster)  [unwired: 3 in, 2 out]
        n135 = invoke on="g2" class="DigNum (strict)" method="Reinit To Default"() -> (error out=w310:errorcluster)  [unwired: 3 in, 2 out]
        n136 = invoke on="w" class="DigNum (strict)" method="Reinit To Default"() -> (error out=w309:errorcluster)  [unwired: 3 in, 2 out]
        n137 = invoke on="q" class="DigNum (strict)" method="Reinit To Default"() -> (error out=w308:errorcluster)  [unwired: 3 in, 2 out]
        n138 = property on="Rotation signal" class="XYGraph (strict)"("Visible"=TRUE) -> (error out=w304:errorcluster)  [unwired: 2 in, 1 out]
        n139 = property on="Rotation signal 3" class="XYGraph (strict)"("Visible"=FALSE) -> (error out=w297:errorcluster)  [unwired: 2 in, 1 out]
        n140 = flat-sequence {
          tunnel: w342 -> [w436]
          tunnel: [w435] -> w340
          frame #0 {
            n141 = Wait (ms)(milliseconds to wait=u32 150) -> ()  [unwired: 1 out]
          }
          frame #1 {
            n142 = invoke on="Run single FID" class="Bool (strict)" method="Reinit To Default"(error in=w436) -> (error out=w435:errorcluster)  [unwired: 2 in, 2 out]
            n143 = local write "Tab Control"(T8."Run single FID" ("Tab Control")) -> ()
          }
        }
        n144 = Concatenate Strings(w356, "\\Zurich_params.ini" ("string")) -> (w349:string)
        n145 = Concatenate Strings(w356, "\\Keithley_params.ini" ("string")) -> (w351:string)
        n146 = Concatenate Strings(w356, "\\pulse_sequence_DAQ.ini" ("string")) -> (w350:string)
        n147 = Bundle By Name(cluster=T7 {"ZI config file (.ini)"="Config_Ver_2\\Zurich_params.ini", "Keithley config file (.ini)"="Config_Ver_2\\Keithley_params.ini", "DAQ config file (.ini)"="Config_Ver_2\\pulse_sequence_DAQ.ini"} ("Config files paths"), "ZI config file (.ini)"=w349, "Keithley config file (.ini)"=w351, "DAQ config file (.ini)"=w350) -> (w346:T7)
        n148 = Merge Errors(w311, w312, w313, w314, w310, w309, w308, w304, w297) -> (w307:errorcluster)
        n149 = Build Array(w303, w303) -> (w302:T12[])
        n150 = call "Initialize_Devices_Main_v2.vi"("error in"=w340, "Resource Address"=w359) -> ("error out"=w357:errorcluster, "Resources"=w358:T13)  [unwired: 8 in]
        n151 = Obtain Queue(name (unnamed)="Data Queue", element data type=w302, error in (no error)=w340) -> (queue out=w339:refnum<queue>, error out=w306:errorcluster)  [unwired: 2 in, 1 out]
        n152 = call "Configurate_All_Main_v2.vi"("Resources in"=w358, "Config files paths"=w346, "error in"=w357) -> ("Resources out"=w348:T13, "error out"=w347:errorcluster)  [unwired: 6 in, 5 out]
        n153 = Merge Errors(w306, w307) -> (w305:errorcluster)
        n154 = for {
          N: "Number of repetition" -> [w426]
          tunnel: w346 -> [w431]
          shift-right: [w430] -> w345
          shift-left: w348 -> [w433]
          shift-right: [w418] -> w344
          shift-left: w347 -> [w432]
          tunnel: w339 -> [w421]
          i -> [w427]
          n155 = Divide(x=w427, y=w426) -> (x/y=w424:dbl)
          n156 = call "Single_Measurement_Main_v2.vi"("Config files paths"=w431, "error in"=w432, "Resources in"=w433) -> ("error out"=w428:errorcluster, "Resources out"=w429:T13)  [unwired: 6 in, 1 out]
          n157 = Multiply(x=w424, y=100.0) -> (x*y=→"Progress":dbl)
          n158 = call "Poll_Data_Main_v2.vi"("error in"=w428, "Resources in"=w429) -> ("error out"=w419:errorcluster, "ZI Data 3"=w420:T12, "ZI Data 0"=w417:T12, "Resources out"=w430:T13)  [unwired: 6 in]
          n159 = Build Array(w417, w420) -> (w422:T12[])
          n160 = Enqueue Element(queue=w421, element=w422, error in (no error)=w419) -> (error out=w418:errorcluster)  [unwired: 1 in, 2 out]
        }
        n161 = call "Close_Devices_Main_v2.vi"("error in"=w344, "Resources"=w345) -> ("error out"=w322:errorcluster)  [unwired: 9 in]
        n162 = Initialize Array(0.0 ("element"), w337) -> (w335:dbl[])
        n163 = for {
          N: "Number of repetition" -> [_]
          tunnel: w339 -> [w410]
          shift-right: [w407] -> w301
          shift-left: w305 -> [w412]
          tunnel: [w410] -> w338
          shift-right: [w400] -> w318
          shift-left: w335 -> [w403]
          tunnel: w337 -> [w406]
          shift-right: [w401] -> w319
          shift-left: w335 -> [w402]
          tunnel: [w389] -> w334
          tunnel: ["Signal in X or Y (?)"] -> w333
          n164 = Dequeue Element(queue=w410, timeout in ms (-1)=10000, error in (no error)=w412) -> (element=w411:T12[], error out=w408:errorcluster)  [unwired: 2 out]
          n165 = Index Array(array=w411) -> (element #1=w391:T12, element #2=w409:T12)  [unwired: 2 in]
          n166 = call "Clear_Data_Main_v2.vi"("ZI Data 0"=w391, "ZI Data 3"=w409, "Time Of Collected Data (ms)"=500.0, 3:"Fixed Number Of Points"=w406, "error in"=w408, 10:"Fixed Number Of Points"=TRUE ("Fixed Number Of Points"), "Check Phase Mismatch"=FALSE) -> ("Cutted Data 0"=w405:T16, "Cutted Data 3"=w404:T16, "error out"=w407:errorcluster)  [unwired: 7 in, 3 out]
          n167 = call "Prepare_plots_SubVI_v1.vi"("Signal in X or Y (?)"="Signal in X or Y (?)", "Y rot avg in"=w402, "X rot avg in"=w403, "Cutted Data 3"=w404, "Cutted Data 0"=w405) -> ("Y rot avg out"=w401:dbl[], "X rot avg out"=w400:dbl[], "Monitor"=→"Intensity signal":cluster{"Time":dbl[], dbl[]}, "RF out"=→"Differential signal":cluster{"Time":dbl[], "Y":dbl[]}[], "Rotation spectrum"=→"Rotation spectrum":waveform(dbl)[], "Rotation"=w396:cluster{"Time":dbl[], dbl[]}[], "Polarimeter"=→"Polarimeter":dbl)
          n168 = Index Array(array=w396) -> (element #1=w395:cluster{"Time":dbl[], dbl[]}, element #2=w394:cluster{"Time":dbl[], dbl[]})  [unwired: 2 in]
          n169 = Select(t=w395, s="Signal in X or Y (?)", f=w394) -> (s? t:f=w389:cluster{"Time":dbl[], dbl[]})
          "Rotation signal" <- w389
        }
        n170 = flat-sequence {
          tunnel: w322 -> [_]
          frame #0 {
            n171 = local write "Progress"(100.0 ("Progress")) -> ()
          }
        }
        n172 = Merge Errors(w322, w301) -> (w300:errorcluster)
        n173 = Divide(x=w318, y="Number of repetition") -> (x/y=w316:dbl[])
        n174 = Divide(x=w319, y="Number of repetition") -> (x/y=w317:dbl[])
        n175 = Unbundle By Name(w334) -> ("Time"=w325:dbl[])
        n176 = Release Queue(queue=w338, error in (no error)=w300) -> (error out=w299:errorcluster)  [unwired: 1 in, 2 out]
        n177 = Build Array(w316, w317) -> (w326:dbl[][])
        n178 = case shown="Error .." w299 {
          selector: w299 -> [w369 w370]
          tunnel: [w369 w373] -> w321
          frame No Error {
          }
          frame Error {
            w378 = "\r\n"
            n179 = Unbundle By Name(w370) -> ("code"=w381:i32, "source"=w379:string)
            n180 = Number To Decimal String(number=w381) -> (decimal integer string=w380:string)  [unwired: 1 in]
            n181 = Concatenate Strings("There is an error:" ("string"), w378, w380, w378, w379, w378, "Do you want to clear it?" ("string")) -> (w374:string)
            n182 = Two Button Dialog(message=w374, 1:"No" ("F button name (\"Cancel\")"), 2:"Yes" ("T button name (\"OK\")")) -> (T button?=w372:bool)
            n183 = call <vilib>:"Clear Errors.vi"("error in (no error)"=w370) -> ("error out"=w371:errorcluster)  [unwired: 5 in, 1 out]
            n184 = Select(t=w371, s=w372, f=w370) -> (s? t:f=w373:errorcluster)
          }
        }
        n185 = Bundle("Time"=w325, w316) -> (w331:cluster{"Time":dbl[], dbl[]})  [unwired: 1 in]
        n186 = Bundle("Time"=w325, w317) -> (w332:cluster{"Time":dbl[], dbl[]})  [unwired: 1 in]
        n187 = Index Array(array=w325, index #1=1 ("index"), index #2=0 ("index")) -> (element #1=w329:dbl, element #2=w330:dbl)
        n188 = Subtract(x=w329, y=w330) -> (x-y=w324:dbl)
        n189 = Select(t=w331, s=w333, f=w332) -> (s? t:f=w295:cluster{"Time":dbl[], dbl[]})
        n190 = local write "Rotation signal"(w295) -> ()
        n191 = for {
          tunnel: w326 -> [w388] mode=indexing
          tunnel: [w386] -> w323 mode=indexing
          tunnel: w324 -> [w383]
          n192 = call <vilib>:"Auto Power Spectrum.vi"("dt"=w383, "Signal (V)"=w388) -> ("df"=w387:dbl, "Power Spectrum (V^2 rms)"=w385:dbl[])
          n193 = Square Root(x=w385) -> (sqrt(x)=w384:dbl[])
          n194 = Bundle By Name("Y"=w384, "dt"=w387) -> (w386:waveform(dbl))  [unwired: 1 in]
        }
        n195 = local read "save"() -> (w296:bool)
        n196 = case shown="True" w296 {
          tunnel: w295 -> [_ w368]
          frame False {
          }
          frame True {
            n197 = Unbundle(w368) -> ("Time"=w367:dbl[], w366:dbl[])
            n198 = Build Array(w367, w366) -> (w365:dbl[][])
            n199 = call <vilib>:"Create File with Incrementing Suffix.vi"("format string (\" (%d)\")"=" %d" ("format string (\" (%d)\")"), "file path"=path "C:/Users/Daniel/Desktop/tests/test.dat") -> ("actual path"=w362:path)  [unwired: 7 in, 2 out]
            n200 = Transpose 2D Array(2D array=w365) -> (transposed array=w364:dbl[][])
            n201 = call-poly <vilib>:"Write Delimited Spreadsheet.vi"("file path (dialog if empty)"=w362, "format (%.3f)"="%.6f", "2D data"=w364) -> ()  [unwired: 11 in, 2 out]
          }
        }
        n202 = local write "Rotation spectrum"(w323) -> ()
      }
      event "Run tomography", "Run tomography 2": Mouse Down {
        w446 = T12 {"R"=[], "Theta"=[], "X"=[], "Y"=[], "AuxIn0"=[], "AuxIn1"=[], "Frequency"=[], "DIO"=[], "Time"=[]} ("ZI Data")
        w441 = "\\tomography" ("string")
        n203 = event-data() -> ()  [unwired: 1 in, 8 out]
        n204 = local read "Config folder"() -> (w442:string)
        n205 = local read "Resource Address"() -> (w471:T3)
        n206 = Build Array(w446, w446) -> (w445:T12[])
        n207 = flat-sequence {
          frame #0 {
            n208 = Wait (ms)(milliseconds to wait=u32 150) -> ()  [unwired: 1 out]
          }
          frame #1 {
            n209 = invoke on="Run tomography" class="Bool (strict)" method="Reinit To Default"() -> ()  [unwired: 3 in, 3 out]
            n210 = local write "Tab Control"(T1."Run tomography" ("Tab Control")) -> ()
          }
        }
        n211 = Concatenate Strings("Config_files\\" ("string"), w442, w441) -> (w444:string)
        n212 = Concatenate Strings(w442, w441, "\\" ("string")) -> (w440:string)
        n213 = call <vilib>:"Application Directory.vi"() -> ("Application Directory"=w474:path)
        n214 = Obtain Queue(name (unnamed)="Data Queue 2", element data type=w445, error in (no error)=w466) -> (queue out=w468:refnum<queue>, error out=w465:errorcluster)  [unwired: 2 in, 1 out]
        n215 = property on="Plot type" class="Ring (strict)"("DisabledEnum"=T9."Disabled and Grayed Out" ("Disabled")) -> (error out=w452:errorcluster)  [unwired: 2 in, 1 out]
        n216 = Concatenate Strings(w442, "\\Zurich_params.ini" ("string")) -> (w477:string)
        n217 = Concatenate Strings(w442, "\\Keithley_params.ini" ("string")) -> (w478:string)
        n218 = Build Path(base path=w474, name or relative path=w444) -> (appended path=w475:path)
        n219 = List Folder(path=w475) -> (filenames=w473:string[])  [unwired: 3 in, 3 out]
        n220 = call "Initialize_Devices_Main_v2.vi"("error in"=w465, "Resource Address"=w471) -> ("error out"=w469:errorcluster, "Resources"=w470:T13)  [unwired: 8 in]
        n221 = for {
          tunnel: "pulses type (priv)" -> [w484] mode=indexing
          tunnel: [w482] -> w455 mode=concatenating
          n222 = for {
            tunnel: " + " ("string") -> [w489]
            tunnel: w484 -> [w488]
            tunnel: string[] ["[ None ]", "[ Y pi ]", "[ Z(pi/2)+Y(pi) ]"] -> [w487] mode=indexing
            tunnel: [w486] -> w482 mode=indexing
            n223 = Concatenate Strings(w488, w489, w487) -> (w486:string)
          }
        }
        n224 = for {
          N -> [w518]
          tunnel: w478 -> [w526]
          tunnel: w477 -> [w525]
          tunnel: w473 -> [w490] mode=indexing
          shift-right: [w521] -> w438
          shift-left: w469 -> [w496]
          tunnel: w468 -> [w522]
          shift-right: [w523] -> w464
          shift-left: w470 -> [w495]
          tunnel: u16 58000 ("Fixed Number Of Points") -> [w519]
          tunnel: [w520] -> w462
          shift-right: [w514] -> w459
          shift-left: dbl[][] [] -> [w515]
          tunnel: w455 -> [_]
          tunnel: [w511] -> w454 mode=indexing
          tunnel: w452 -> [_]
          tunnel: w440 -> [w492]
          i -> [w512]
          n225 = Concatenate Strings(w492, w490) -> (w491:string)
          n226 = Multiply(x="Averaging", y=w512) -> (x*y=w517:i32)
          n227 = Bundle By Name(cluster=T7 {"ZI config file (.ini)"="Config_Ver_2\\Zurich_params.ini", "Keithley config file (.ini)"="Config_Ver_2\\Keithley_params.ini", "DAQ config file (.ini)"="Config_Ver_2\\pulse_sequence_DAQ.ini"} ("Config files paths"), "ZI config file (.ini)"=w525, "Keithley config file (.ini)"=w526, "DAQ config file (.ini)"=w491) -> (w493:T7)
          n228 = call "Configurate_All_Main_v2.vi"("Resources in"=w495, "Config files paths"=w493, "error in"=w496) -> ("Resources out"=w494:T13, "error out"=w497:errorcluster)  [unwired: 6 in, 5 out]
          n229 = for {
            N: "Averaging" -> [w575]
            shift-right: [w587] -> w523
            shift-left: w494 -> [w589]
            shift-right: [w578] -> w509
            shift-left: w497 -> [w588]
            tunnel: w522 -> [w580]
            tunnel: w493 -> [w577]
            tunnel: w518 -> [w576]
            tunnel: w517 -> [w572]
            i -> [w573]
            n230 = Add(x=w573, y=w572) -> (x+y=w571:i32)
            n231 = Multiply(x=w575, y=w576) -> (x*y=w574:i32)
            n232 = call "Single_Measurement_Main_v2.vi"("Config files paths"=w577, "error in"=w588, "Resources in"=w589) -> ("error out"=w585:errorcluster, "Resources out"=w586:T13)  [unwired: 6 in, 1 out]
            n233 = call "Poll_Data_Main_v2.vi"("error in"=w585, "Resources in"=w586) -> ("error out"=w579:errorcluster, "ZI Data 3"=w582:T12, "ZI Data 0"=w569:T12, "Resources out"=w587:T13)  [unwired: 6 in]
            n234 = Divide(x=w571, y=w574) -> (x/y=w583:dbl)
            n235 = Build Array(w569, w582) -> (w581:T12[])
            n236 = Multiply(x=w583, y=100.0) -> (x*y=→"Progress":dbl)
            n237 = Enqueue Element(queue=w580, element=w581, error in (no error)=w579) -> (error out=w578:errorcluster)  [unwired: 1 in, 2 out]
          }
          n238 = Initialize Array(0.0 ("element"), w519) -> (w506:dbl[])
          n239 = for {
            N: "Averaging" -> [_]
            shift-right: [w560] -> w510
            shift-left: w496 -> [w565]
            shift-right: [w554] -> w504
            shift-left: w506 -> [w557]
            shift-right: [w555] -> w505
            shift-left: w506 -> [w556]
            tunnel: [w547] -> w500
            tunnel: w522 -> [w546]
            tunnel: w519 -> [w545]
            tunnel: [w544] -> w502
            n240 = local read "Signal in X or Y (?)"() -> (w547:bool)
            n241 = Dequeue Element(queue=w546, timeout in ms (-1)=10000, error in (no error)=w565) -> (element=w564:T12[], error out=w561:errorcluster)  [unwired: 2 out]
            n242 = Index Array(array=w564) -> (element #1=w562:T12, element #2=w563:T12)  [unwired: 2 in]
            n243 = call "Clear_Data_Main_v2.vi"("ZI Data 0"=w562, "ZI Data 3"=w563, "Time Of Collected Data (ms)"=500.0, 3:"Fixed Number Of Points"=w545, "error in"=w561, 10:"Fixed Number Of Points"=TRUE ("Fixed Number Of Points"), "Check Phase Mismatch"=FALSE) -> ("Cutted Data 0"=w559:T16, "Cutted Data 3"=w558:T16, "error out"=w560:errorcluster)  [unwired: 7 in, 3 out]
            n244 = call "Prepare_plots_SubVI_v1.vi"("Signal in X or Y (?)"=w547, "Y rot avg in"=w556, "X rot avg in"=w557, "Cutted Data 3"=w558, "Cutted Data 0"=w559) -> ("Y rot avg out"=w555:dbl[], "X rot avg out"=w554:dbl[], "Monitor"=→"Intensity signal":cluster{"Time":dbl[], dbl[]}, "RF out"=→"Differential signal":cluster{"Time":dbl[], "Y":dbl[]}[], "Rotation spectrum"=→"Rotation spectrum":waveform(dbl)[], "Rotation"=w551:cluster{"Time":dbl[], dbl[]}[])  [unwired: 1 out]
            n245 = Index Array(array=w551) -> (element #1=w550:cluster{"Time":dbl[], dbl[]}, element #2=w549:cluster{"Time":dbl[], dbl[]})  [unwired: 2 in]
            n246 = Select(t=w550, s=w547, f=w549) -> (s? t:f=w544:cluster{"Time":dbl[], dbl[]})
            "Rotation signal" <- w544
          }
          n247 = Divide(x=w504, y="Averaging") -> (x/y=w498:dbl[])
          n248 = Divide(x=w505, y="Averaging") -> (x/y=w499:dbl[])
          n249 = Empty Array?(array=w515) -> (empty?=w503:bool)
          n250 = Unbundle By Name(w502) -> ("Time"=w501:dbl[])
          n251 = Merge Errors(w509, w510) -> (w508:errorcluster)
          n252 = case shown="True" w503 {
            tunnel: w501 -> [w528 w535]
            tunnel: w515 -> [w534 w542]
            tunnel: [w533 w541] -> w514
            tunnel: w500 -> [w532 w540]
            tunnel: w499 -> [w531 w539]
            tunnel: w498 -> [w530 w538]
            tunnel: [w527 w537] -> w513
            frame True {
              n253 = Select(t=w530, s=w532, f=w531) -> (s? t:f=w529:dbl[])
              n254 = Bundle("Time"=w528, w529) -> (w527:cluster{"Time":dbl[], dbl[]})  [unwired: 1 in]
              n255 = Build Array (concatenate)(w534, w528, w529) -> (w533:dbl[][])
            }
            frame False {
              n256 = Select(t=w538, s=w540, f=w539) -> (s? t:f=w536:dbl[])
              n257 = Bundle("Time"=w535, w536) -> (w537:cluster{"Time":dbl[], dbl[]})  [unwired: 1 in]
              n258 = Build Array (concatenate)(w542, w536) -> (w541:dbl[][])
            }
          }
          n259 = Flush Queue(queue=w522, error in (no error)=w508) -> (queue out=w520:refnum<queue>, error out=w521:errorcluster)  [unwired: 1 out]
          n260 = flat-sequence {
            tunnel: w513 -> [w590]
            tunnel: w512 -> [w591]
            tunnel: [w590] -> w511
            frame #0 {
              n261 = local write "Plot type"(w591) -> ()
              "Rotation" <- w590
            }
          }
        }
        "tomography rotation memory (priv)" <- w454
        n262 = property on="Plot type" class="Ring (strict)"("Strings []"=w455) -> ()  [unwired: 2 in, 2 out]
        n263 = Release Queue(queue=w462, error in (no error)=w438) -> (error out=w461:errorcluster)  [unwired: 1 in, 2 out]
        n264 = flat-sequence {
          tunnel: w438 -> [_]
          frame #0 {
            n265 = local write "Progress"(100.0 ("Progress")) -> ()
          }
        }
        n266 = call "Close_Devices_Main_v2.vi"("error in"=w461, "Resources"=w464) -> ("error out"=w450:errorcluster)  [unwired: 9 in]
        n267 = property on="Plot type" class="Ring (strict)"(error in=w438, "DisabledEnum"=T9."Enabled" ("Disabled")) -> (error out=w449:errorcluster)  [unwired: 1 in, 1 out]
        n268 = call "Save_Tomography_Data_Main_v2.vi"("error in"=w438, "Save CYCLOPS data (?)"="Save CYCLOPS data (?)", "Save raw data (?)"="Save raw data (?)", "Data Raw"=w459) -> ("error out"=w448:errorcluster)  [unwired: 6 in, 1 out]
        n269 = Merge Errors(w450, w449, w448) -> (w447:errorcluster)
        n270 = case shown="Error .." w447 {
          selector: w447 -> [w592 w593]
          tunnel: [w592 w596] -> w476
          frame No Error {
          }
          frame Error {
            w601 = "\r\n"
            n271 = Unbundle By Name(w593) -> ("code"=w604:i32, "source"=w602:string)
            n272 = Number To Decimal String(number=w604) -> (decimal integer string=w603:string)  [unwired: 1 in]
            n273 = Concatenate Strings("There is an error:" ("string"), w601, w603, w601, w602, w601, "Do you want to clear it?" ("string")) -> (w597:string)
            n274 = Two Button Dialog(message=w597, 1:"No" ("F button name (\"Cancel\")"), 2:"Yes" ("T button name (\"OK\")")) -> (T button?=w595:bool)
            n275 = call <vilib>:"Clear Errors.vi"("error in (no error)"=w593) -> ("error out"=w594:errorcluster)  [unwired: 5 in, 1 out]
            n276 = Select(t=w594, s=w595, f=w593) -> (s? t:f=w596:errorcluster)
          }
        }
      }
      event "Plot type": Value Change {
        n277 = event-data() -> ()  [unwired: 1 in, 6 out]
        n278 = local read "tomography rotation memory (priv)"() -> (w610:cluster{"Time":dbl[], dbl[]}[])
        n279 = local read "Plot type"() -> (w611:u16)
        n280 = Index Array(array=w610, index=w611) -> (element=w612:cluster{"Time":dbl[], dbl[]})
        n281 = local write "Rotation"(w612) -> ()
      }
      event "Fit model": Mouse Down {
        w618 = 2.0 ("x")
        w636 = 5 ("y")
        w643 = 1 ("index")
        # "q"
        # "w"
        # "g"
        # "C"
        # "B"
        # "A"
        # "initial values:"
        n282 = event-data() -> ()  [unwired: 1 in, 8 out]
        n283 = local read "Rotation signal"() -> (w637:cluster{"Time":dbl[], dbl[]})
        n284 = Decrement(x=w643) -> (x-1=w645:i32)
        n285 = Unbundle(w637) -> ("Time"=w644:dbl[], w641:dbl[])
        n286 = property on="Rotation signal" class="XYGraph (strict)"(error in=w651, "Visible"=FALSE) -> (error out=w649:errorcluster)  [unwired: 1 in, 1 out]
        n287 = property on="Rotation signal 3" class="XYGraph (strict)"(error in=w651, "Visible"=TRUE) -> (error out=w650:errorcluster)  [unwired: 1 in, 1 out]
        n288 = local read "Polarimeter"() -> (w626:dbl)
        n289 = Array Size(array=w641) -> (size(s)=w642:i32)
        n290 = Index Array(array=w644, index #1=w643, index #2=w645) -> (element #1=w646:dbl, element #2=w647:dbl)
        n291 = Multiply(x=1100.0, y=6.283185307179586) -> (x*y=w622:dbl)
        n292 = Subtract(x=w646, y=w647) -> (x-y=w635:dbl)
        n293 = Quotient & Remainder(x=w642, y=w636) -> (floor(x/y)=w640:i32)  [unwired: 1 out]
        n294 = Merge Errors(w649, w650) -> (w648:errorcluster)
        n295 = Reshape Array(w641, w640, w636) -> (w639:dbl[][])
        n296 = Multiply(x=w635, y=w636) -> (x*y=w633:dbl)
        n297 = Index Array(array=w639, index (col)=0 ("disabled index (col)")) -> (element=w615:dbl[])  [unwired: 1 in]
        n298 = Array Subset(array=w615, index=0, length=100) -> (w629:dbl[])
        n299 = Array Max & Min(array=w629) -> (max value=w628:dbl, min value=w627:dbl)  [unwired: 2 out]
        n300 = Subtract(x=w628, y=w627) -> (x-y=w619:dbl)
        n301 = Add(x=w628, y=w627) -> (x+y=w620:dbl)
        n302 = Divide(x=w620, y=w618) -> (x/y=w617:dbl)
        n303 = Divide(x=w619, y=w618) -> (x/y=w616:dbl)
        n304 = Array Size(array=w615) -> (size(s)=w634:i32)
        n305 = for {
          N: w634 -> [_]
          tunnel: w633 -> [w659]
          tunnel: [w658] -> w632 mode=indexing
          i -> [w660]
          n306 = Multiply(x=w659, y=w660) -> (x*y=w658:dbl)
        }
        n307 = Multiply(x=w615, y=1000) -> (x*y=w613:dbl[])
        n308 = case shown="\"Full\"" "Enum" {
          tunnel: [w692 w718 w745] -> w654
          tunnel: [w681 w708 w737] -> w652
          tunnel: w648 -> [w681 w708 w737]
          tunnel: w637 -> [w691 w717 w744]
          tunnel: w632 -> [w684 w711 w740]
          tunnel: w617 -> [w690 _ w723]
          tunnel: w626 -> [w689 w716 w722]
          tunnel: 20.0 -> [w688 w715 w721]
          tunnel: w622 -> [_ w702 w720]
          tunnel: 0.0 -> [_ w703 w719]
          tunnel: w616 -> [_ w704 w724]
          tunnel: w613 -> [w685 w712 w741]
          frame "B*Exp(-q2*t)+C" {
            w693 = nan
            n309 = Build Array(w690, w689, w688) -> (w682:dbl[])
            n310 = call-poly <vilib>:"Nonlinear Curve Fit.vi"("Y"=w685, "initial parameters"=w682, "X"=w684, "model description"=T10 {"model"="b*exp(-g2*t)+c", "Parameters"=["b", "c", "g2"], "x"="t"}, "error in (no error)"=w681) -> ("best nonlinear fit"=w683:dbl[], "best fit parameters"=w679:dbl[])  [unwired: 6 in, 3 out]
            n311 = Divide(x=w683, y=1000) -> (x/y=w687:dbl[])
            n312 = Index Array(array=w679) -> (element #1=w678:dbl, element #2=w677:dbl, element #3=w676:dbl)  [unwired: 3 in]
            n313 = Bundle(w684, w687) -> (w675:cluster{dbl[], dbl[]})  [unwired: 1 in]
            n314 = Build Array(w691, w675) -> (w692:cluster{"Time":dbl[], dbl[]}[])
            n315 = local write "A"(w693) -> ()
            n316 = local write "C"(w677) -> ()
            n317 = local write "g2"(w676) -> ()
            n318 = local write "q"(w693) -> ()
            n319 = local write "w"(w693) -> ()
            n320 = local write "g1"(w693) -> ()
            n321 = local write "B"(w678) -> ()
          }
          frame "A*Sin(w*t+q)*Exp(-g1*t)+C" {
            w701 = nan
            n322 = Build Array(w704, w716, w715, w703, w702) -> (w709:dbl[])
            n323 = call-poly <vilib>:"Nonlinear Curve Fit.vi"("Y"=w712, "initial parameters"=w709, "X"=w711, "model description"=T10 {"model"="a*sin(w*t+q)*exp(-g1*t)+c", "Parameters"=["a", "c", "g1", "q", "w"], "x"="t"}, "error in (no error)"=w708) -> ("best nonlinear fit"=w710:dbl[], "best fit parameters"=w706:dbl[])  [unwired: 6 in, 3 out]
            n324 = Divide(x=w710, y=1000) -> (x/y=w714:dbl[])
            n325 = Index Array(array=w706) -> (element #1=w700:dbl, element #2=w699:dbl, element #3=w698:dbl, element #4=w696:dbl, element #5=w697:dbl)  [unwired: 5 in]
            n326 = Bundle(w711, w714) -> (w705:cluster{dbl[], dbl[]})  [unwired: 1 in]
            n327 = Quotient & Remainder(x=w696, y=6.283185307179586) -> (x-y*floor(x/y)=w694:dbl)  [unwired: 1 out]
            n328 = Build Array(w717, w705) -> (w718:cluster{"Time":dbl[], dbl[]}[])
            n329 = local write "g1"(w698) -> ()
            n330 = local write "w"(w697) -> ()
            n331 = local write "A"(w700) -> ()
            n332 = local write "C"(w699) -> ()
            n333 = local write "q"(w694) -> ()
            n334 = local write "B"(w701) -> ()
            n335 = local write "g2"(w701) -> ()
          }
          frame "Full" {
            n336 = Build Array(w724, w723, w722, w721, w721, w720, w719) -> (w738:dbl[])
            n337 = call-poly <vilib>:"Nonlinear Curve Fit.vi"("Y"=w741, "initial parameters"=w738, "X"=w740, "model description"=T10 {"model"="a*sin(w*t+q)*exp(-g1*t)+b*exp(-g2*t)+c", "Parameters"=["a", "b", "c", "g1", "g2", "w", "q"], "x"="t"}, "error in (no error)"=w737) -> ("best nonlinear fit"=w739:dbl[], "best fit parameters"=w728:dbl[])  [unwired: 6 in, 3 out]
            n338 = Divide(x=w739, y=1000) -> (x/y=w743:dbl[])
            n339 = Index Array(array=w728) -> (element #1=w734:dbl, element #2=w730:dbl, element #3=w731:dbl, element #4=w732:dbl, element #5=w733:dbl, element #6=w729:dbl, element #7=w725:dbl)  [unwired: 7 in]
            n340 = Bundle(w740, w743) -> (w735:cluster{dbl[], dbl[]})  [unwired: 1 in]
            n341 = local write "w"(w729) -> ()
            n342 = local write "A"(w734) -> ()
            n343 = local write "B"(w730) -> ()
            n344 = local write "C"(w731) -> ()
            n345 = local write "g1"(w732) -> ()
            n346 = local write "g2"(w733) -> ()
            n347 = Quotient & Remainder(x=w725, y=6.283185307179586) -> (x-y*floor(x/y)=w726:dbl)  [unwired: 1 out]
            n348 = Build Array(w744, w735) -> (w745:cluster{"Time":dbl[], dbl[]}[])
            n349 = local write "q"(w726) -> ()
          }
        }
        n350 = Reverse 1D Array(array=w654) -> (reversed array=→"Rotation signal 3":cluster{"Time":dbl[], dbl[]}[])
        n351 = case shown="Error .." w652 {
          selector: w652 -> [w661 w662]
          tunnel: [w661 w665] -> _
          frame No Error {
          }
          frame Error {
            w670 = "\r\n"
            n352 = Unbundle By Name(w662) -> ("code"=w673:i32, "source"=w671:string)
            n353 = Number To Decimal String(number=w673) -> (decimal integer string=w672:string)  [unwired: 1 in]
            n354 = Concatenate Strings("There is an error:" ("string"), w670, w672, w670, w671, w670, "Do you want to clear it?" ("string")) -> (w666:string)
            n355 = Two Button Dialog(message=w666, 1:"No" ("F button name (\"Cancel\")"), 2:"Yes" ("T button name (\"OK\")")) -> (T button?=w664:bool)
            n356 = call <vilib>:"Clear Errors.vi"("error in (no error)"=w662) -> ("error out"=w663:errorcluster)  [unwired: 5 in, 1 out]
            n357 = Select(t=w663, s=w664, f=w662) -> (s? t:f=w665:errorcluster)
          }
        }
      }
      event "X pi": Mouse Down {
        n358 = event-data() -> ()  [unwired: 1 in, 8 out]
        n359 = Look In Map(map=w751, key="X pi") -> (value=w747:dbl)  [unwired: 1 in, 1 out]
        n360 = Look In Map(map=w751, key="Delay") -> (value=w746:dbl)  [unwired: 1 in, 1 out]
        n361 = Look In Map(map=w757, key="pulse X") -> (value=w748:i32)  [unwired: 1 in, 1 out]
        n362 = Wait (ms)(milliseconds to wait=u32 150) -> ()  [unwired: 1 out]
        n363 = call "Add_to_sequence_SubVI_v1.vi"("Delay [us]"=w746, "Pulse length [us]"=w747, "Channel number"=w748, "Array sequence in"=w750) -> ("Array sequence out"=w749:cluster{"Timing 0":dbl[]}[])
      }
      event "X pi/2": Mouse Down {
        n364 = event-data() -> ()  [unwired: 1 in, 8 out]
        n365 = Look In Map(map=w763, key="X pi/2") -> (value=w759:dbl)  [unwired: 1 in, 1 out]
        n366 = Look In Map(map=w763, key="Delay") -> (value=w758:dbl)  [unwired: 1 in, 1 out]
        n367 = Look In Map(map=w769, key="pulse X") -> (value=w760:i32)  [unwired: 1 in, 1 out]
        n368 = Wait (ms)(milliseconds to wait=u32 150) -> ()  [unwired: 1 out]
        n369 = call "Add_to_sequence_SubVI_v1.vi"("Delay [us]"=w758, "Pulse length [us]"=w759, "Channel number"=w760, "Array sequence in"=w762) -> ("Array sequence out"=w761:cluster{"Timing 0":dbl[]}[])
      }
      event "Y pi": Mouse Down {
        n370 = event-data() -> ()  [unwired: 1 in, 8 out]
        n371 = Look In Map(map=w775, key="Y pi") -> (value=w771:dbl)  [unwired: 1 in, 1 out]
        n372 = Look In Map(map=w775, key="Delay") -> (value=w770:dbl)  [unwired: 1 in, 1 out]
        n373 = Look In Map(map=w781, key="pulse Y") -> (value=w772:i32)  [unwired: 1 in, 1 out]
        n374 = Wait (ms)(milliseconds to wait=u32 150) -> ()  [unwired: 1 out]
        n375 = call "Add_to_sequence_SubVI_v1.vi"("Delay [us]"=w770, "Pulse length [us]"=w771, "Channel number"=w772, "Array sequence in"=w774) -> ("Array sequence out"=w773:cluster{"Timing 0":dbl[]}[])
      }
      event "Y pi/2": Mouse Down {
        n376 = event-data() -> ()  [unwired: 1 in, 8 out]
        n377 = Look In Map(map=w787, key="Y pi/2") -> (value=w783:dbl)  [unwired: 1 in, 1 out]
        n378 = Look In Map(map=w787, key="Delay") -> (value=w782:dbl)  [unwired: 1 in, 1 out]
        n379 = Look In Map(map=w793, key="pulse Y") -> (value=w784:i32)  [unwired: 1 in, 1 out]
        n380 = Wait (ms)(milliseconds to wait=u32 150) -> ()  [unwired: 1 out]
        n381 = call "Add_to_sequence_SubVI_v1.vi"("Delay [us]"=w782, "Pulse length [us]"=w783, "Channel number"=w784, "Array sequence in"=w786) -> ("Array sequence out"=w785:cluster{"Timing 0":dbl[]}[])
      }
      event "Z pi": Mouse Down {
        n382 = event-data() -> ()  [unwired: 1 in, 8 out]
        n383 = Look In Map(map=w799, key="Z pi") -> (value=w795:dbl)  [unwired: 1 in, 1 out]
        n384 = Look In Map(map=w799, key="Delay") -> (value=w794:dbl)  [unwired: 1 in, 1 out]
        n385 = Look In Map(map=w805, key="pulse Z") -> (value=w796:i32)  [unwired: 1 in, 1 out]
        n386 = Wait (ms)(milliseconds to wait=u32 150) -> ()  [unwired: 1 out]
        n387 = call "Add_to_sequence_SubVI_v1.vi"("Delay [us]"=w794, "Pulse length [us]"=w795, "Channel number"=w796, "Array sequence in"=w798) -> ("Array sequence out"=w797:cluster{"Timing 0":dbl[]}[])
      }
      event "Z pi/2": Mouse Down {
        n388 = event-data() -> ()  [unwired: 1 in, 8 out]
        n389 = Look In Map(map=w811, key="Z pi/2") -> (value=w807:dbl)  [unwired: 1 in, 1 out]
        n390 = Look In Map(map=w811, key="Delay") -> (value=w806:dbl)  [unwired: 1 in, 1 out]
        n391 = Look In Map(map=w817, key="pulse Z") -> (value=w808:i32)  [unwired: 1 in, 1 out]
        n392 = Wait (ms)(milliseconds to wait=u32 150) -> ()  [unwired: 1 out]
        n393 = call "Add_to_sequence_SubVI_v1.vi"("Delay [us]"=w806, "Pulse length [us]"=w807, "Channel number"=w808, "Array sequence in"=w810) -> ("Array sequence out"=w809:cluster{"Timing 0":dbl[]}[])
      }
      event "Add pulse": Mouse Down {
        n394 = event-data() -> ()  [unwired: 1 in, 8 out]
        n395 = Index Array(array=w829, index="Channel") -> (element=w827:string)
        n396 = Look In Map(map=w823, key="Delay") -> (value=w818:dbl)  [unwired: 1 in, 1 out]
        n397 = Look In Map(map=w828, key=w827) -> (value=w820:i32)  [unwired: 1 in, 1 out]
        n398 = call "Add_to_sequence_SubVI_v1.vi"("Delay [us]"=w818, "Pulse length [us]"="Time [us]", "Channel number"=w820, "Array sequence in"=w822) -> ("Array sequence out"=w821:cluster{"Timing 0":dbl[]}[])
        n399 = Wait (ms)(milliseconds to wait=u32 150) -> ()  [unwired: 1 out]
      }
      event "Add pulse advanced": Mouse Down {
        # "Search for choosen channels"
        n400 = event-data() -> ()  [unwired: 1 in, 8 out]
        n401 = for {
          tunnel: "Physical channels" -> [w850] mode=indexing
          tunnel: w843 -> [w851]
          tunnel: [w849] -> w842 mode=indexing
          tunnel: [w847] -> w839 mode=indexing
          n402 = Search 1D Array(1D array=w851, element=w850) -> (index of element=w849:i32)  [unwired: 1 in]
          n403 = Equal?(x=w849, y=-1) -> (x = y?=w847:bool)
        }
        n404 = Or Array Elements(Boolean array=w839) -> (logical OR=w838:bool)
        n405 = case shown="True" w838 {
          frame False {
          }
          frame True {
            n406 = One Button Dialog(message="Some port names are not correct!!!\nPulse sequance may not be correct!") -> ()  [unwired: 1 in, 1 out]
          }
        }
        n407 = for {
          tunnel: w845 -> [w853] mode=indexing
          tunnel: w842 -> [w857]
          tunnel: [w852] -> w835 mode=indexing
          i -> [w856]
          n408 = for {
            tunnel: w857 -> [w873] mode=indexing
            tunnel: w856 -> [w874]
            tunnel: [w872] -> w855 mode=indexing
            n409 = Equal?(x=w873, y=w874) -> (x = y?=w872:bool)
          }
          n410 = Or Array Elements(Boolean array=w855) -> (logical OR=w854:bool)
          n411 = case shown="True" w854 {
            tunnel: w853 -> [w860 w867]
            tunnel: [w858 w865] -> w852
            frame True {
              n412 = local read "Time [us]"() -> (w859:dbl)
              n413 = in-place {
                in-place-border: w859 -> [w863]
                n414 = in-place-cluster #9(w860) -> ("Timing 0"=w864:dbl[])
                n415 = Build Array (concatenate)(w864, w863, 0.0 ("element")) -> (w861:dbl[])
                n416 = in-place-cluster #9("Timing 0"=w861) -> (w858:cluster{"Timing 0":dbl[]})
              }
            }
            frame False {
              n417 = local read "Time [us]"() -> (w866:dbl)
              n418 = in-place {
                in-place-border: w866 -> [w869]
                n419 = in-place-cluster #10(w867) -> ("Timing 0"=w871:dbl[])
                n420 = Build Array (concatenate)(w871, 0.0 ("element"), w869) -> (w870:dbl[])
                n421 = in-place-cluster #10("Timing 0"=w870) -> (w865:cluster{"Timing 0":dbl[]})
              }
            }
          }
        }
        n422 = Look In Map(map=w837, key="Delay") -> (value=w831:dbl)  [unwired: 1 in, 1 out]
        n423 = Wait (ms)(milliseconds to wait=u32 150) -> ()  [unwired: 1 out]
        n424 = call "Add_to_sequence_SubVI_v1.vi"("Delay [us]"=w831, "Pulse length [us]"=0.0, "Channel number"=-1, "Array sequence in"=w835) -> ("Array sequence out"=w834:cluster{"Timing 0":dbl[]}[])
      }
      event "Save single sequence": Mouse Down {
        n425 = event-data() -> ()  [unwired: 1 in, 8 out]
        n426 = Look In Map(map=w897, key="Accqusition TRIG") -> (value=w887:i32)  [unwired: 1 in, 1 out]
        n427 = Look In Map(map=w894, key="TTL") -> (value=w886:dbl)  [unwired: 1 in, 1 out]
        n428 = Look In Map(map=w894, key="Delay") -> (value=w885:dbl)  [unwired: 1 in, 1 out]
        n429 = Look In Map(map=w894, key="Probe") -> (value=w889:dbl)  [unwired: 1 in, 1 out]
        n430 = for {
          tunnel: w884 -> [w906] mode=indexing
          tunnel: w886 -> [w905]
          tunnel: [w904] -> w888 mode=indexing
          tunnel: w887 -> [w903]
          i -> [w902]
          n431 = Equal?(x=w903, y=w902) -> (x = y?=w907:bool)
          n432 = case shown="True" w907 {
            tunnel: w906 -> [w908 w911]
            tunnel: w905 -> [_ w910]
            tunnel: [w908 w909] -> w904
            frame False {
            }
            frame True {
              n433 = in-place {
                in-place-border: w910 -> [w912]
                n434 = in-place-cluster #11(w911) -> ("Timing 0"=w913:dbl[])
                n435 = Build Array (concatenate)(w913, w912) -> (w914:dbl[])
                n436 = in-place-cluster #11("Timing 0"=w914) -> (w909:cluster{"Timing 0":dbl[]})
              }
            }
          }
        }
        n437 = Look In Map(map=w897, key="Keithley TRIG") -> (value=w892:i32)  [unwired: 1 in, 1 out]
        n438 = for {
          tunnel: w888 -> [w935] mode=indexing
          tunnel: w892 -> [w937]
          tunnel: w886 -> [w934]
          tunnel: w885 -> [w933]
          tunnel: [w932] -> w890 mode=indexing
          i -> [w938]
          n439 = Equal?(x=w938, y=w937) -> (x = y?=w936:bool)
          n440 = case shown="True" w936 {
            tunnel: w935 -> [w939 w943]
            tunnel: w934 -> [_ w942]
            tunnel: w933 -> [_ w941]
            tunnel: [w939 w940] -> w932
            frame False {
            }
            frame True {
              n441 = in-place {
                in-place-border: w942 -> [w947]
                in-place-border: w941 -> [w946]
                n442 = in-place-cluster #12(w943) -> ("Timing 0"=w949:dbl[])
                n443 = Multiply(x=2.0, y=w946) -> (x*y=w944:dbl)
                n444 = Build Array (concatenate)(w949, 0.0, w944, w947) -> (w950:dbl[])
                n445 = in-place-cluster #12("Timing 0"=w950) -> (w940:cluster{"Timing 0":dbl[]})
              }
            }
          }
        }
        n446 = Look In Map(map=w897, key="LD probe") -> (value=w891:i32)  [unwired: 1 in, 1 out]
        n447 = flat-sequence {
          frame #0 {
            n448 = Wait (ms)(milliseconds to wait=u32 150) -> ()  [unwired: 1 out]
          }
          frame #1 {
            n449 = invoke on="Save single sequence" class="Bool (strict)" method="Reinit To Default"() -> ()  [unwired: 3 in, 3 out]
          }
        }
        n450 = for {
          tunnel: w891 -> [w920]
          tunnel: w890 -> [w918] mode=indexing
          tunnel: w889 -> [w917]
          tunnel: [w916] -> w883 mode=indexing
          tunnel: w885 -> [w915]
          i -> [w921]
          n451 = Equal?(x=w921, y=w920) -> (x = y?=w919:bool)
          n452 = case shown="True" w919 {
            tunnel: w918 -> [w922 w926]
            tunnel: [w922 w925] -> w916
            tunnel: w917 -> [_ w924]
            tunnel: w915 -> [_ w923]
            frame False {
            }
            frame True {
              n453 = in-place {
                in-place-border: w924 -> [w927]
                in-place-border: w923 -> [w928]
                n454 = in-place-cluster #13(w926) -> ("Timing 0"=w930:dbl[])
                n455 = Build Array (concatenate)(w930, 0.0, w928, w927) -> (w931:dbl[])
                n456 = in-place-cluster #13("Timing 0"=w931) -> (w925:cluster{"Timing 0":dbl[]})
              }
            }
          }
        }
        n457 = call "Array_to_cluster_sequence_SubVI_v1.vi"("Array"=w883) -> ("Sequence"=w882:T6)
        n458 = local read "Sampling data"() -> (w880:T2)
        n459 = local read "Config folder"() -> (w877:string)
        n460 = Concatenate Strings(w877, "\\pulse_sequence_DAQ.ini" ("string")) -> (w875:string)
        n461 = call "Set_Pulse_Seq_DAQ.vi"("Time Unit"=T11 {"Time Unit"=enum."MicroSecond"}, "error in"=w879, "Sampling data"=w880, "Sequence"=w882, "Filename (ini)"=w875) -> ("error out"=w878:errorcluster)  [unwired: 6 in]
      }
      event "Save for tomography": Mouse Down {
        w957 = string[][] [["None", "None"], ["Y pi", "None"], ["Z pi/2", "Y pi"]]
        w951 = string[] ["None", "Y pi/2", "X pi/2"]
        # "Additional delay to ensure that\nall measurement start at the\nsame moment"
        # "CYCLOPS"
        # "Control pulses"
        n462 = event-data() -> ()  [unwired: 1 in, 8 out]
        n463 = local write "pulses type (priv)"(w951) -> ()
        n464 = for {
          tunnel: w959 -> [w1087]
          tunnel: w951 -> [w1086] mode=indexing
          tunnel: [w1085] -> w966 mode=indexing
          # "Check longest control pulse"
          n465 = Look In Map(map=w1087, key=w1086) -> (value=w1085:dbl)  [unwired: 1 in, 1 out]
        }
        n466 = Look In Map(map=w959, key="Delay") -> (value=w964:dbl)  [unwired: 1 in, 1 out]
        n467 = for {
          tunnel: w959 -> [w1093]
          tunnel: w957 -> [w1092] mode=indexing
          tunnel: w964 -> [w1089]
          tunnel: [w1088] -> w965 mode=indexing
          # "Check longest CYCLOPS sequence"
          n468 = for {
            tunnel: w1093 -> [w1096]
            tunnel: [w1095] -> w1091 mode=indexing
            tunnel: w1092 -> [w1094] mode=indexing
            n469 = Look In Map(map=w1096, key=w1094) -> (value=w1095:dbl)  [unwired: 1 in, 1 out]
          }
          n470 = Add Array Elements(numeric array=w1091) -> (sum=w1090:dbl)
          n471 = Add(x=w1090, y=w1089) -> (x+y=w1088:dbl)
        }
        n472 = for {
          tunnel: w966 -> [w1083] mode=indexing
          tunnel: w965 -> [w1084]
          tunnel: w964 -> [w1081]
          tunnel: [w1082] -> w962 mode=indexing
          n473 = Compound Arithmetic op=unknown(w1084, w1081, w1083, w1081) -> (w1082:dbl[])
        }
        n474 = Array Max & Min(array=w962) -> (max value=w963:dbl)  [unwired: 3 out]
        n475 = Subtract(x=w963, y=w962) -> (x-y=w956:dbl[][])
        n476 = for {
          tunnel: string[] ["None", "pulse Y", "pulse X"] -> [w993] mode=indexing
          tunnel: w951 -> [w994] mode=indexing
          tunnel: w955 -> [w995]
          tunnel: w960 -> [w984]
          tunnel: w959 -> [w985]
          tunnel: string[][] [["None", "None"], ["pulse Y", "None"], ["pulse Z", "pulse Y"]] -> [w988]
          tunnel: w957 -> [w987]
          tunnel: [w983] -> w954 mode=concatenating
          tunnel: w956 -> [w982] mode=indexing
          # "Iterate over control pulses"
          n477 = Look In Map(map=w984, key=w993) -> (value=w991:i32)  [unwired: 1 in, 1 out]
          n478 = Look In Map(map=w985, key=w994) -> (value=w990:dbl)  [unwired: 1 in, 1 out]
          n479 = Look In Map(map=w985, key="Delay") -> (value=w986:dbl)  [unwired: 1 in, 1 out]
          n480 = call "Add_to_sequence_SubVI_v1.vi"("Delay [us]"=w986, "Pulse length [us]"=w990, "Channel number"=w991, "Array sequence in"=w995) -> ("Array sequence out"=w989:cluster{"Timing 0":dbl[]}[])
          n481 = for {
            tunnel: w989 -> [w1022]
            tunnel: w988 -> [w1019] mode=indexing
            tunnel: w987 -> [w1020] mode=indexing
            tunnel: w986 -> [w1021]
            tunnel: w985 -> [w1004]
            tunnel: w984 -> [w1000]
            tunnel: [w1003] -> w983 mode=indexing
            tunnel: w982 -> [w998] mode=indexing
            # "Add equalization of the time interval"
            # "Iterate over CYCLOPS in 2 for loops because CYCLOPS consists of a few pulses"
            n482 = for {
              shift-right: [w1073] -> w1002
              shift-left: w1022 -> [w1076]
              tunnel: w1021 -> [w1072]
              tunnel: w1020 -> [w1079] mode=indexing
              tunnel: w1019 -> [w1080] mode=indexing
              tunnel: w1004 -> [w1078]
              tunnel: w1000 -> [w1077]
              tunnel: [w1072] -> w997
              n483 = Look In Map(map=w1077, key=w1080) -> (value=w1075:i32)  [unwired: 1 in, 1 out]
              n484 = Look In Map(map=w1078, key=w1079) -> (value=w1074:dbl)  [unwired: 1 in, 1 out]
              n485 = call "Add_to_sequence_SubVI_v1.vi"("Delay [us]"=w1072, "Pulse length [us]"=w1074, "Channel number"=w1075, "Array sequence in"=w1076) -> ("Array sequence out"=w1073:cluster{"Timing 0":dbl[]}[])
            }
            n486 = Look In Map(map=w1000, key="None") -> (value=w999:i32)  [unwired: 1 in, 1 out]
            n487 = call "Add_to_sequence_SubVI_v1.vi"("Delay [us]"=w997, "Pulse length [us]"=w998, "Channel number"=w999, "Array sequence in"=w1002) -> ("Array sequence out"=w996:cluster{"Timing 0":dbl[]}[])
            n488 = Look In Map(map=w1004, key="Probe") -> (value=w1014:dbl)  [unwired: 1 in, 1 out]
            n489 = Look In Map(map=w1004, key="Delay") -> (value=w1018:dbl)  [unwired: 1 in, 1 out]
            n490 = Look In Map(map=w1000, key="Accqusition TRIG") -> (value=w1016:i32)  [unwired: 1 in, 1 out]
            n491 = Look In Map(map=w1004, key="TTL") -> (value=w1017:dbl)  [unwired: 1 in, 1 out]
            n492 = for {
              tunnel: w996 -> [w1027] mode=indexing
              tunnel: w1017 -> [w1026]
              tunnel: [w1025] -> w1015 mode=indexing
              tunnel: w1016 -> [w1024]
              i -> [w1023]
              n493 = Equal?(x=w1024, y=w1023) -> (x = y?=w1028:bool)
              n494 = case shown="True" w1028 {
                tunnel: w1027 -> [w1029 w1032]
                tunnel: w1026 -> [_ w1031]
                tunnel: [w1029 w1030] -> w1025
                frame False {
                }
                frame True {
                  n495 = in-place {
                    in-place-border: w1031 -> [w1033]
                    n496 = in-place-cluster #14(w1032) -> ("Timing 0"=w1034:dbl[])
                    n497 = Build Array (concatenate)(w1034, w1033) -> (w1035:dbl[])
                    n498 = in-place-cluster #14("Timing 0"=w1035) -> (w1030:cluster{"Timing 0":dbl[]})
                  }
                }
              }
            }
            n499 = Look In Map(map=w1000, key="Keithley TRIG") -> (value=w1011:i32)  [unwired: 1 in, 1 out]
            n500 = for {
              tunnel: w1015 -> [w1056] mode=indexing
              tunnel: w1011 -> [w1058]
              tunnel: w1017 -> [w1055]
              tunnel: w1018 -> [w1054]
              tunnel: [w1053] -> w1013 mode=indexing
              i -> [w1059]
              n501 = Equal?(x=w1059, y=w1058) -> (x = y?=w1057:bool)
              n502 = case shown="True" w1057 {
                tunnel: w1056 -> [w1060 w1064]
                tunnel: w1055 -> [_ w1063]
                tunnel: w1054 -> [_ w1062]
                tunnel: [w1060 w1061] -> w1053
                frame False {
                }
                frame True {
                  n503 = in-place {
                    in-place-border: w1063 -> [w1068]
                    in-place-border: w1062 -> [w1067]
                    n504 = in-place-cluster #15(w1064) -> ("Timing 0"=w1070:dbl[])
                    n505 = Multiply(x=2.0, y=w1067) -> (x*y=w1065:dbl)
                    n506 = Build Array (concatenate)(w1070, 0.0, w1065, w1068) -> (w1071:dbl[])
                    n507 = in-place-cluster #15("Timing 0"=w1071) -> (w1061:cluster{"Timing 0":dbl[]})
                  }
                }
              }
            }
            n508 = Look In Map(map=w1000, key="LD probe") -> (value=w1012:i32)  [unwired: 1 in, 1 out]
            n509 = for {
              tunnel: w1012 -> [w1041]
              tunnel: w1013 -> [w1039] mode=indexing
              tunnel: w1014 -> [w1038]
              tunnel: [w1037] -> w1003 mode=indexing
              tunnel: w1018 -> [w1036]
              i -> [w1042]
              n510 = Equal?(x=w1042, y=w1041) -> (x = y?=w1040:bool)
              n511 = case shown="True" w1040 {
                tunnel: w1039 -> [w1043 w1047]
                tunnel: [w1043 w1046] -> w1037
                tunnel: w1038 -> [_ w1045]
                tunnel: w1036 -> [_ w1044]
                frame False {
                }
                frame True {
                  n512 = in-place {
                    in-place-border: w1045 -> [w1048]
                    in-place-border: w1044 -> [w1049]
                    n513 = in-place-cluster #16(w1047) -> ("Timing 0"=w1051:dbl[])
                    n514 = Build Array (concatenate)(w1051, 0.0, w1049, w1048) -> (w1052:dbl[])
                    n515 = in-place-cluster #16("Timing 0"=w1052) -> (w1046:cluster{"Timing 0":dbl[]})
                  }
                }
              }
            }
          }
        }
        n516 = flat-sequence {
          frame #0 {
            n517 = Wait (ms)(milliseconds to wait=u32 150) -> ()  [unwired: 1 out]
          }
          frame #1 {
            n518 = invoke on="Save for tomography" class="Bool (strict)" method="Reinit To Default"() -> ()  [unwired: 3 in, 3 out]
          }
        }
        n519 = for {
          tunnel: w954 -> [w981] mode=indexing
          shift-right: [w969] -> w952
          shift-left: w953 -> [w979]
          i -> [w974]
          n520 = local read "Config folder"() -> (w976:string)
          n521 = Number To Decimal String(number=w974, width (-)=i16 1) -> (decimal integer string=w972:string)
          n522 = call "Array_to_cluster_sequence_SubVI_v1.vi"("Array"=w981) -> ("Sequence"=w980:T6)
          n523 = local read "Sampling data"() -> (w978:T2)
          n524 = Concatenate Strings(w976, "\\tomography\\pulse_seq_DAQ_" ("string"), w972, ".ini" ("string")) -> (w970:string)
          n525 = call "Set_Pulse_Seq_DAQ.vi"("Time Unit"=T11 {"Time Unit"=enum."MicroSecond"}, "error in"=w979, "Sampling data"=w978, "Sequence"=w980, "Filename (ini)"=w970) -> ("error out"=w969:errorcluster)  [unwired: 6 in]
        }
      }
      event "Reset sequence": Mouse Down {
        n526 = event-data() -> ()  [unwired: 1 in, 8 out]
        n527 = Wait (ms)(milliseconds to wait=u32 150) -> ()  [unwired: 1 out]
      }
    }
  }
